vi "Thermal_Camera_Calibration.vi"() -> (2 "State out":string="Data: Load Thermal Calibration")   [LabVIEW 2020]
uses:
  DataCluster_TCAL.ctl
  <vilib>/vision/Image Controls.llb/IMAQ Image.ctl
  DataCluster.ctl
  <vilib>/userdefined/High Color/IMAQdx.ctl
  <vilib>/Utility/xml.llb/Write to XML File(string).vi
panel:
  out "Pict Ring":i32(ring)
  in  "Done":bool
  out "Step":string="Step: 4\n\nCalculate temperature!"
  in  "Fixpoint Radius":i32=20 min=3 max=20
  in  "Cluster":T1 {"PCR Size" items=["384 (24x16)", "96 (12x8)"]; "Points"."Top Left"."Y" format="%.2f"; "Points"."Top Left"."X" format="%.2f"; "Points"."Top Right"."Y" format="%.2f"; "Points"."Top Right"."X" format="%.2f"; "Points"."Bottom Left"."Y" format="%.2f"; "Points"."Bottom Left"."X" format="%.2f"; "Points"."Bottom Right"."Y" format="%.2f"; "Points"."Bottom Right"."X" format="%.2f"; "Points"."Fixpoint"."Y" format="%.2f"; "Points"."Fixpoint"."X" format="%.2f"}
  in  "Display Mapping":u32(ring)=10 items=["Default"=10, "Most Significant Bits"=11, "Full Dynamic"=12, "Downshift"=13, "Given Range"=14, "90% Dynamic"=15, "Given Percent Range"=16]
  in  "Image":u32(slide) scale=0.0..242.0
  in  "Help":bool
  out "Tutorial":string="Step: 4\n\nCalculate temperature!"
  in  "Show All Points":bool
  in  "Well Radius":u32=50 min=1 max=100
  in  "PCR Size":u16(ring) items=["384 (24x16)", "96 (12x8)"]
  out "Points":T3[](array[typedef])=[{"X"=103.0, "Y"=94.0}, {"X"=158.04349, "Y"=93.521736}, {"X"=213.08696, "Y"=93.04348}, {"X"=268.13043, "Y"=92.565216}, {"X"=323.17392, "Y"=92.08696}, {"X"=378.2174, "Y"=91.608696}, {"X"=433.26086, "Y"=91.13043}, {"X"=488.30435, "Y"=90.652176}, {"X"=543.34784, "Y"=90.17391}, {"X"=598.39136, "Y"=89.69565}, {"X"=653.4348, "Y"=89.21739}, {"X"=708.4783, "Y"=88.73913}, {"X"=763.5217, "Y"=88.26087}, {"X"=818.56525, "Y"=87.78261}, {"X"=873.6087, "Y"=87.30435}, {"X"=928.6522, "Y"=86.82609}, {"X"=983.6957, "Y"=86.347824}, {"X"=1038.7391, "Y"=85.86957}, {"X"=1093.7827, "Y"=85.391304}, {"X"=1148.8262, "Y"=84.91304}, {"X"=1203.8696, "Y"=84.434784}, {"X"=1258.9131, "Y"=83.95652}, {"X"=1313.9565, "Y"=83.478264}, {"X"=1369.0, "Y"=83.0}, {"X"=103.46667, "Y"=149.06667}, {"X"=158.51015, "Y"=148.58841}, {"X"=213.55362, "Y"=148.11014}, {"X"=268.5971, "Y"=147.63188}, {"X"=323.6406, "Y"=147.15363}, {"X"=378.68408, "Y"=146.67535}, {"X"=433.72754, "Y"=146.1971}, {"X"=488.77103, "Y"=145.71884}, {"X"=543.8145, "Y"=145.24057}, {"X"=598.858, "Y"=144.76231}, {"X"=653.9015, "Y"=144.28406}, {"X"=708.94495, "Y"=143.8058}, {"X"=763.9884, "Y"=143.32753}, {"X"=819.0319, "Y"=142.84927}, {"X"=874.0754, "Y"=142.37102}, {"X"=929.1189, "Y"=141.89276}, {"X"=984.16235, "Y"=141.41449}, {"X"=1039.2058, "Y"=140.93623}, {"X"=1094.2493, "Y"=140.45798}, {"X"=1149.2928, "Y"=139.9797}, {"X"=1204.3363, "Y"=139.50145}, {"X"=1259.3798, "Y"=139.0232}, {"X"=1314.4232, "Y"=138.54492}, {"X"=1369.4667, "Y"=138.06667}, {"X"=103.933334, "Y"=204.13333}, {"X"=158.9768, "Y"=203.65506}, {"X"=214.0203, "Y"=203.17682}, {"X"=269.06375, "Y"=202.69855}, {"X"=324.10724, "Y"=202.22029}, {"X"=379.15073, "Y"=201.74203}, {"X"=434.19418, "Y"=201.26376}, {"X"=489.23767, "Y"=200.7855}, {"X"=544.2812, "Y"=200.30725}, {"X"=599.32465, "Y"=199.82898}, {"X"=654.36816, "Y"=199.35072}, {"X"=709.4116, "Y"=198.87247}, {"X"=764.4551, "Y"=198.3942}, {"X"=819.4986, "Y"=197.91594}, {"X"=874.54205, "Y"=197.43768}, {"X"=929.5856, "Y"=196.95941}, {"X"=984.629, "Y"=196.48116}, {"X"=1039.6725, "Y"=196.0029}, {"X"=1094.716, "Y"=195.52463}, {"X"=1149.7595, "Y"=195.04637}, {"X"=1204.803, "Y"=194.56812}, {"X"=1259.8464, "Y"=194.08984}, {"X"=1314.8899, "Y"=193.6116}, {"X"=1369.9333, "Y"=193.13333}, {"X"=104.4, "Y"=259.2}, {"X"=159.44348, "Y"=258.72174}, {"X"=214.48695, "Y"=258.24347}, {"X"=269.53043, "Y"=257.7652}, {"X"=324.5739, "Y"=257.28696}, {"X"=379.6174, "Y"=256.8087}, {"X"=434.66086, "Y"=256.33044}, {"X"=489.70435, "Y"=255.85217}, {"X"=544.74786, "Y"=255.37392}, {"X"=599.7913, "Y"=254.89565}, {"X"=654.83484, "Y"=254.41739}, {"X"=709.8783, "Y"=253.93913}, {"X"=764.92175, "Y"=253.46086}, {"X"=819.9653, "Y"=252.9826}, {"X"=875.0087, "Y"=252.50435}, {"X"=930.05225, "Y"=252.02608}, {"X"=985.0957, "Y"=251.54782}, {"X"=1040.1392, "Y"=251.06956}, {"X"=1095.1826, "Y"=250.59131}, {"X"=1150.2262, "Y"=250.11304}, {"X"=1205.2697, "Y"=249.63478}, {"X"=1260.3131, "Y"=249.15652}, {"X"=1315.3566, "Y"=248.67825}, {"X"=1370.4, "Y"=248.2}, {"X"=104.86667, "Y"=314.26666}, {"X"=159.91014, "Y"=313.7884}, {"X"=214.95363, "Y"=313.31012}, {"X"=269.9971, "Y"=312.83188}, {"X"=325.0406, "Y"=312.35364}, {"X"=380.08408, "Y"=311.87537}, {"X"=435.12753, "Y"=311.3971}, {"X"=490.17102, "Y"=310.91882}, {"X"=545.2145, "Y"=310.44058}, {"X"=600.258, "Y"=309.9623}, {"X"=655.30145, "Y"=309.48407}, {"X"=710.3449, "Y"=309.0058}, {"X"=765.38837, "Y"=308.52753}, {"X"=820.4319, "Y"=308.04926}, {"X"=875.47534, "Y"=307.571}, {"X"=930.51886, "Y"=307.09274}, {"X"=985.5623, "Y"=306.6145}, {"X"=1040.6058, "Y"=306.13623}, {"X"=1095.6493, "Y"=305.65796}, {"X"=1150.6929, "Y"=305.1797}, {"X"=1205.7363, "Y"=304.70145}, {"X"=1260.7798, "Y"=304.2232}, {"X"=1315.8232, "Y"=303.74493}, {"X"=1370.8667, "Y"=303.26666}, {"X"=105.333336, "Y"=369.3333}, {"X"=160.37682, "Y"=368.85504}, {"X"=215.42029, "Y"=368.3768}, {"X"=270.46378, "Y"=367.89853}, {"X"=325.50726, "Y"=367.42026}, {"X"=380.55075, "Y"=366.94202}, {"X"=435.5942, "Y"=366.46375}, {"X"=490.6377, "Y"=365.98547}, {"X"=545.68115, "Y"=365.50723}, {"X"=600.7247, "Y"=365.02896}, {"X"=655.7681, "Y"=364.5507}, {"X"=710.8116, "Y"=364.07245}, {"X"=765.85504, "Y"=363.59418}, {"X"=820.89856, "Y"=363.11594}, {"X"=875.942, "Y"=362.63766}, {"X"=930.98553, "Y"=362.1594}, {"X"=986.029, "Y"=361.68115}, {"X"=1041.0725, "Y"=361.20288}, {"X"=1096.116, "Y"=360.7246}, {"X"=1151.1595, "Y"=360.24637}, {"X"=1206.203, "Y"=359.7681}, {"X"=1261.2465, "Y"=359.28983}, {"X"=1316.2899, "Y"=358.81158}, {"X"=1371.3334, "Y"=358.3333}, {"X"=105.8, "Y"=424.4}, {"X"=160.84348, "Y"=423.92172}, {"X"=215.88696, "Y"=423.44348}, {"X"=270.93042, "Y"=422.9652}, {"X"=325.9739, "Y"=422.48694}, {"X"=381.0174, "Y"=422.0087}, {"X"=436.06085, "Y"=421.53043}, {"X"=491.10434, "Y"=421.05215}, {"X"=546.1478, "Y"=420.5739}, {"X"=601.19135, "Y"=420.09564}, {"X"=656.2348, "Y"=419.61737}, {"X"=711.27826, "Y"=419.13913}, {"X"=766.3217, "Y"=418.66086}, {"X"=821.36523, "Y"=418.18262}, {"X"=876.4087, "Y"=417.70435}, {"X"=931.4522, "Y"=417.22607}, {"X"=986.49567, "Y"=416.74783}, {"X"=1041.5392, "Y"=416.26956}, {"X"=1096.5826, "Y"=415.7913}, {"X"=1151.6262, "Y"=415.31305}, {"X"=1206.6697, "Y"=414.83478}, {"X"=1261.7131, "Y"=414.3565}, {"X"=1316.7566, "Y"=413.87827}, {"X"=1371.8, "Y"=413.4}, {"X"=106.26667, "Y"=479.46667}, {"X"=161.31015, "Y"=478.9884}, {"X"=216.35362, "Y"=478.51016}, {"X"=271.3971, "Y"=478.0319}, {"X"=326.44058, "Y"=477.55362}, {"X"=381.48407, "Y"=477.07538}, {"X"=436.52753, "Y"=476.5971}, {"X"=491.571, "Y"=476.11884}, {"X"=546.6145, "Y"=475.6406}, {"X"=601.658, "Y"=475.16232}, {"X"=656.7015, "Y"=474.68405}, {"X"=711.74493, "Y"=474.2058}, {"X"=766.7884, "Y"=473.72754}, {"X"=821.8319, "Y"=473.2493}, {"X"=876.87537, "Y"=472.77103}, {"X"=931.9189, "Y"=472.29276}, {"X"=986.96234, "Y"=471.8145}, {"X"=1042.0059, "Y"=471.33624}, {"X"=1097.0493, "Y"=470.85797}, {"X"=1152.0929, "Y"=470.37973}, {"X"=1207.1364, "Y"=469.90146}, {"X"=1262.1798, "Y"=469.4232}, {"X"=1317.2233, "Y"=468.94495}, {"X"=1372.2667, "Y"=468.46667}, {"X"=106.73333, "Y"=534.5333}, {"X"=161.77681, "Y"=534.05505}, {"X"=216.8203, "Y"=533.5768}, {"X"=271.86377, "Y"=533.0985}, {"X"=326.90726, "Y"=532.62024}, {"X"=381.95074, "Y"=532.142}, {"X"=436.9942, "Y"=531.66376}, {"X"=492.0377, "Y"=531.1855}, {"X"=547.0812, "Y"=530.7073}, {"X"=602.12463, "Y"=530.229}, {"X"=657.16815, "Y"=529.75073}, {"X"=712.2116, "Y"=529.27246}, {"X"=767.25507, "Y"=528.7942}, {"X"=822.2986, "Y"=528.3159}, {"X"=877.34204, "Y"=527.83765}, {"X"=932.38556, "Y"=527.3594}, {"X"=987.429, "Y"=526.88116}, {"X"=1042.4724, "Y"=526.4029}, {"X"=1097.516, "Y"=525.9246}, {"X"=1152.5594, "Y"=525.4464}, {"X"=1207.6029, "Y"=524.96814}, {"X"=1262.6464, "Y"=524.48987}, {"X"=1317.6898, "Y"=524.0116}, {"X"=1372.7333, "Y"=523.5333}, {"X"=107.2, "Y"=589.6}, {"X"=162.24348, "Y"=589.1217}, {"X"=217.28696, "Y"=588.64343}, {"X"=272.33044, "Y"=588.16516}, {"X"=327.37393, "Y"=587.6869}, {"X"=382.41742, "Y"=587.2087}, {"X"=437.46088, "Y"=586.7304}, {"X"=492.50436, "Y"=586.25214}, {"X"=547.54785, "Y"=585.7739}, {"X"=602.5913, "Y"=585.29565}, {"X"=657.6348, "Y"=584.8174}, {"X"=712.6783, "Y"=584.3391}, {"X"=767.72174, "Y"=583.86084}, {"X"=822.76526, "Y"=583.38257}, {"X"=877.8087, "Y"=582.9043}, {"X"=932.85223, "Y"=582.426}, {"X"=987.8957, "Y"=581.9478}, {"X"=1042.9391, "Y"=581.46954}, {"X"=1097.9827, "Y"=580.9913}, {"X"=1153.0261, "Y"=580.51306}, {"X"=1208.0696, "Y"=580.0348}, {"X"=1263.113, "Y"=579.5565}, {"X"=1318.1565, "Y"=579.07825}, {"X"=1373.2, "Y"=578.6}, {"X"=107.666664, "Y"=644.6666}, {"X"=162.71014, "Y"=644.18835}, {"X"=217.75363, "Y"=643.7101}, {"X"=272.7971, "Y"=643.2319}, {"X"=327.84058, "Y"=642.7536}, {"X"=382.88406, "Y"=642.2753}, {"X"=437.92752, "Y"=641.79706}, {"X"=492.971, "Y"=641.3188}, {"X"=548.0145, "Y"=640.8405}, {"X"=603.058, "Y"=640.3623}, {"X"=658.1015, "Y"=639.88403}, {"X"=713.14496, "Y"=639.40576}, {"X"=768.1884, "Y"=638.9275}, {"X"=823.23193, "Y"=638.4492}, {"X"=878.2754, "Y"=637.97095}, {"X"=933.3189, "Y"=637.49274}, {"X"=988.36237, "Y"=637.01447}, {"X"=1043.4058, "Y"=636.5362}, {"X"=1098.4493, "Y"=636.0579}, {"X"=1153.4928, "Y"=635.57965}, {"X"=1208.5363, "Y"=635.1014}, {"X"=1263.5797, "Y"=634.62317}, {"X"=1318.6232, "Y"=634.1449}, {"X"=1373.6666, "Y"=633.6666}, {"X"=108.13333, "Y"=699.73334}, {"X"=163.17682, "Y"=699.25507}, {"X"=218.22029, "Y"=698.7768}, {"X"=273.26376, "Y"=698.2986}, {"X"=328.30725, "Y"=697.8203}, {"X"=383.35074, "Y"=697.34204}, {"X"=438.3942, "Y"=696.8638}, {"X"=493.43768, "Y"=696.3855}, {"X"=548.4812, "Y"=695.9072}, {"X"=603.52466, "Y"=695.429}, {"X"=658.5682, "Y"=694.95074}, {"X"=713.61163, "Y"=694.4725}, {"X"=768.6551, "Y"=693.9942}, {"X"=823.6986, "Y"=693.5159}, {"X"=878.74207, "Y"=693.03766}, {"X"=933.7856, "Y"=692.55945}, {"X"=988.82904, "Y"=692.0812}, {"X"=1043.8724, "Y"=691.6029}, {"X"=1098.916, "Y"=691.12463}, {"X"=1153.9595, "Y"=690.64636}, {"X"=1209.0029, "Y"=690.1681}, {"X"=1264.0464, "Y"=689.6899}, {"X"=1319.0898, "Y"=689.2116}, {"X"=1374.1333, "Y"=688.73334}, {"X"=108.6, "Y"=754.8}, {"X"=163.64348, "Y"=754.3217}, {"X"=218.68697, "Y"=753.84344}, {"X"=273.73044, "Y"=753.36523}, {"X"=328.77393, "Y"=752.88696}, {"X"=383.8174, "Y"=752.4087}, {"X"=438.86087, "Y"=751.9304}, {"X"=493.90436, "Y"=751.45215}, {"X"=548.9478, "Y"=750.9739}, {"X"=603.99133, "Y"=750.49567}, {"X"=659.0348, "Y"=750.0174}, {"X"=714.07825, "Y"=749.5391}, {"X"=769.1217, "Y"=749.06085}, {"X"=824.1652, "Y"=748.5826}, {"X"=879.2087, "Y"=748.1043}, {"X"=934.2522, "Y"=747.6261}, {"X"=989.29565, "Y"=747.1478}, {"X"=1044.3391, "Y"=746.66956}, {"X"=1099.3827, "Y"=746.1913}, {"X"=1154.4261, "Y"=745.713}, {"X"=1209.4696, "Y"=745.23474}, {"X"=1264.5131, "Y"=744.75653}, {"X"=1319.5565, "Y"=744.27826}, {"X"=1374.6, "Y"=743.8}, {"X"=109.066666, "Y"=809.86664}, {"X"=164.11015, "Y"=809.38837}, {"X"=219.15363, "Y"=808.9101}, {"X"=274.1971, "Y"=808.4319}, {"X"=329.2406, "Y"=807.9536}, {"X"=384.2841, "Y"=807.47534}, {"X"=439.32755, "Y"=806.9971}, {"X"=494.37103, "Y"=806.5188}, {"X"=549.4145, "Y"=806.0405}, {"X"=604.458, "Y"=805.5623}, {"X"=659.50146, "Y"=805.08405}, {"X"=714.5449, "Y"=804.6058}, {"X"=769.5884, "Y"=804.1275}, {"X"=824.6319, "Y"=803.64923}, {"X"=879.67535, "Y"=803.17096}, {"X"=934.7189, "Y"=802.69275}, {"X"=989.7623, "Y"=802.2145}, {"X"=1044.8058, "Y"=801.7362}, {"X"=1099.8494, "Y"=801.25793}, {"X"=1154.8928, "Y"=800.77966}, {"X"=1209.9363, "Y"=800.3014}, {"X"=1264.9797, "Y"=799.8232}, {"X"=1320.0232, "Y"=799.3449}, {"X"=1375.0667, "Y"=798.86664}, {"X"=109.53333, "Y"=864.93335}, {"X"=164.57681, "Y"=864.4551}, {"X"=219.6203, "Y"=863.9768}, {"X"=274.66376, "Y"=863.4986}, {"X"=329.70724, "Y"=863.0203}, {"X"=384.75073, "Y"=862.54205}, {"X"=439.7942, "Y"=862.0638}, {"X"=494.83768, "Y"=861.5855}, {"X"=549.88116, "Y"=861.10724}, {"X"=604.9247, "Y"=860.629}, {"X"=659.96814, "Y"=860.15076}, {"X"=715.0116, "Y"=859.6725}, {"X"=770.05505, "Y"=859.1942}, {"X"=825.0986, "Y"=858.71594}, {"X"=880.142, "Y"=858.2377}, {"X"=935.18555, "Y"=857.75946}, {"X"=990.229, "Y"=857.2812}, {"X"=1045.2725, "Y"=856.8029}, {"X"=1100.316, "Y"=856.32465}, {"X"=1155.3595, "Y"=855.8464}, {"X"=1210.403, "Y"=855.3681}, {"X"=1265.4464, "Y"=854.8899}, {"X"=1320.4899, "Y"=854.4116}, {"X"=1375.5333, "Y"=853.93335}, {"X"=110.0, "Y"=920.0}, {"X"=165.04349, "Y"=919.5217}, {"X"=220.08696, "Y"=919.04346}, {"X"=275.13043, "Y"=918.56525}, {"X"=330.17392, "Y"=918.087}, {"X"=385.2174, "Y"=917.6087}, {"X"=440.26086, "Y"=917.13043}, {"X"=495.30435, "Y"=916.65216}, {"X"=550.34784, "Y"=916.1739}, {"X"=605.39136, "Y"=915.6957}, {"X"=660.4348, "Y"=915.2174}, {"X"=715.4783, "Y"=914.73914}, {"X"=770.5217, "Y"=914.26086}, {"X"=825.56525, "Y"=913.7826}, {"X"=880.6087, "Y"=913.3043}, {"X"=935.6522, "Y"=912.8261}, {"X"=990.6957, "Y"=912.34784}, {"X"=1045.7391, "Y"=911.86957}, {"X"=1100.7827, "Y"=911.3913}, {"X"=1155.8262, "Y"=910.913}, {"X"=1210.8696, "Y"=910.43475}, {"X"=1265.9131, "Y"=909.95654}, {"X"=1320.9565, "Y"=909.4783}, {"X"=1376.0, "Y"=909.0}] {"Y" format="%.2f"; "X" format="%.2f"}
  out "State":i32=3
  in  "Previous":bool
  in  "Next":bool
  in  "Path":path caption="Image Path"
  out "Image":T2(plugin-control)
  # "hints \nPress F1 or F2 to cycle through the steps\nUse the Mouse Wheel to zoom in and out"
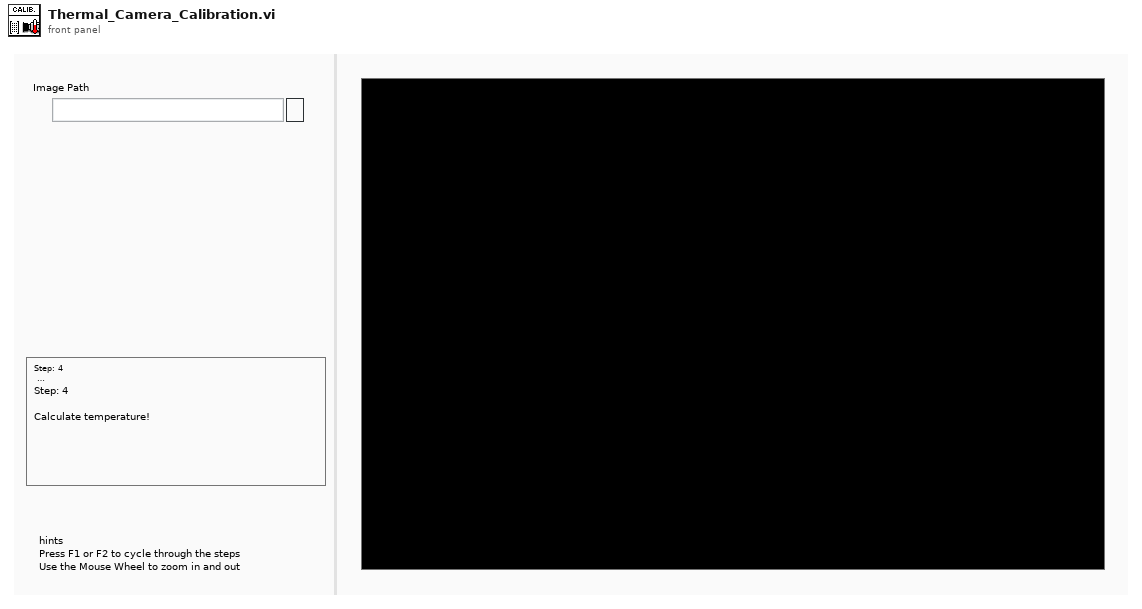
[diagram p1: front panel]
types:
  T1 = typedef "DataCluster_TCAL.ctl" = cluster{"Core":cluster{"Current VI Reference":refnum<vi>, "Close Panel on Exit?":bool}, "Image Out":T2, "State":i32, "Points":cluster{"Top Left":T3, "Top Right":T3, "Bottom Left":T3, "Bottom Right":T3, "x space 2":dbl, "y space 2":sgl, "x_space":sgl, "y_space":sgl, "Pixels":cluster{"X":i32, "Y":i32}[][], "Fixpoint":T3}, "img_array":T2[], "Temps":dbl[], "Temps_Array":dbl[][], "Scan Area":dbl, "Fixpoint Area":dbl, "PCR Size":u16}
  T2 = typedef "IMAQ Image.ctl" = refnum<image>
  T3 = typedef "IMAQ Point" = cluster{"X":sgl, "Y":sgl}
  T4 = enum32{"Invalid", "Standard", "Closed", "Hidden", "Minimized", "Maximized"}
  T5 = enum32{"invalid app kind", "Development System", "Run Time System", "Student Edition", "Embedded LabVIEW", "Evaluation", "Custom"}
  T6 = cluster{"Global Rectangle":i32[], "Contours":cluster{"Contour Type":u32, "ROI Type":u32, "Points":i32[]}[]}
  T7 = typedef "DataCluster.ctl" = cluster{"Core":cluster{"Current VI Reference":refnum<vi>, "Close Panel on Exit?":bool, "Exit":bool, "Initialized?":bool}, "Connections":cluster{"cDAQ Therm":cluster{"Task":refnum<k21>, "Connected":bool, "Active":bool}, "cDAQ Voltage":cluster{"Task":refnum<k21>, "Connected":bool, "Active":bool}, "cDAQ ID":string, "Camera":cluster{"Session":T8, "Connected":bool, "Active":bool, "Placeholder":T2}, "PSU":cluster{"Port":refnum<visa-resource-name>, "Connected":bool, "Active":bool}}, "Data Acquisition":cluster{"Setup":cluster{"Label":string, "Operator":string, "Notes":string, "TempGrad":dbl, "TargetTemp":dbl, "Sample Volume":dbl}, "Camera":cluster{"Image":T2, "Save Image":T2, "Image Frequency":i32, "Rectangle":T9, "Calibration":cluster{"Top Left":T3, "Top Right":T3, "Bottom Left":T3, "Bottom Right":T3, "Fixpoint":T3, "Scan Area":dbl, "Fixpoint Area":dbl, "Well Pixels":cluster{"X":i32, "Y":i32}[][], "Valid":bool}, "FocusPos":u32, "Display Mapping":u32}, "Thermistor":cluster{"Sample Size":i32, "Calibration":cluster{"B0.100":dbl[], "R25":dbl[], "c":dbl[][], "State":bool[], "V_S":dbl, "R_S":dbl}, "Timing Mode":i32}, "Partition":cluster{"Data":string[][], "Cell Label":string, "Cell Color":u32, "Height":i32, "Width":i32, "Grid":string[][]}, "Queue":cluster{"Size":i32, "Queue":refnum<queue>}, "Sample Rate":i32, "Active":bool, "Ready":bool, "Graph Mode":u16}, "Control":cluster{"Sample Rate":i32, "PID gains":cluster{"proportional gain (Kc)":dbl, "integral time (Ti, min)":dbl, "derivative time (Td, min)":dbl}}}
  T8 = typedef "IMAQdx.ctl" = refnum<k21>
  T9 = typedef "IMAQ Rectangle" = cluster{"Left":i32, "Top":i32, "Right":i32, "Bottom":i32, "Rotation":dbl}
  T10 = enum16{"open", "replace", "create", "open or create", "replace or create", "replace or create with confirmation"}
  T11 = typedef "ROI Descriptor" = cluster{"Global Rectangle":i32[], "Contours":cluster{"ID":enum32{"External", "Internal"}, "Type":u32, "Coordinates":i32[]}[]}
  T12 = typedef "Image Type" = u32
  T13 = cluster{"Current VI Reference":refnum<vi>, "Close Panel on Exit?":bool}
  T14 = cluster{"Top Left":T3, "Top Right":T3, "Bottom Left":T3, "Bottom Right":T3, "x space 2":dbl, "y space 2":sgl, "x_space":sgl, "y_space":sgl, "Pixels":cluster{"X":i32, "Y":i32}[][], "Fixpoint":T3}
  T15 = cluster{"Top Left":T3, "Top Right":T3, "Bottom Left":T3, "Bottom Right":T3, "Fixpoint":T3, "Scan Area":dbl, "Fixpoint Area":dbl, "Well Pixels":cluster{"X":i32, "Y":i32}[][], "Valid":bool}
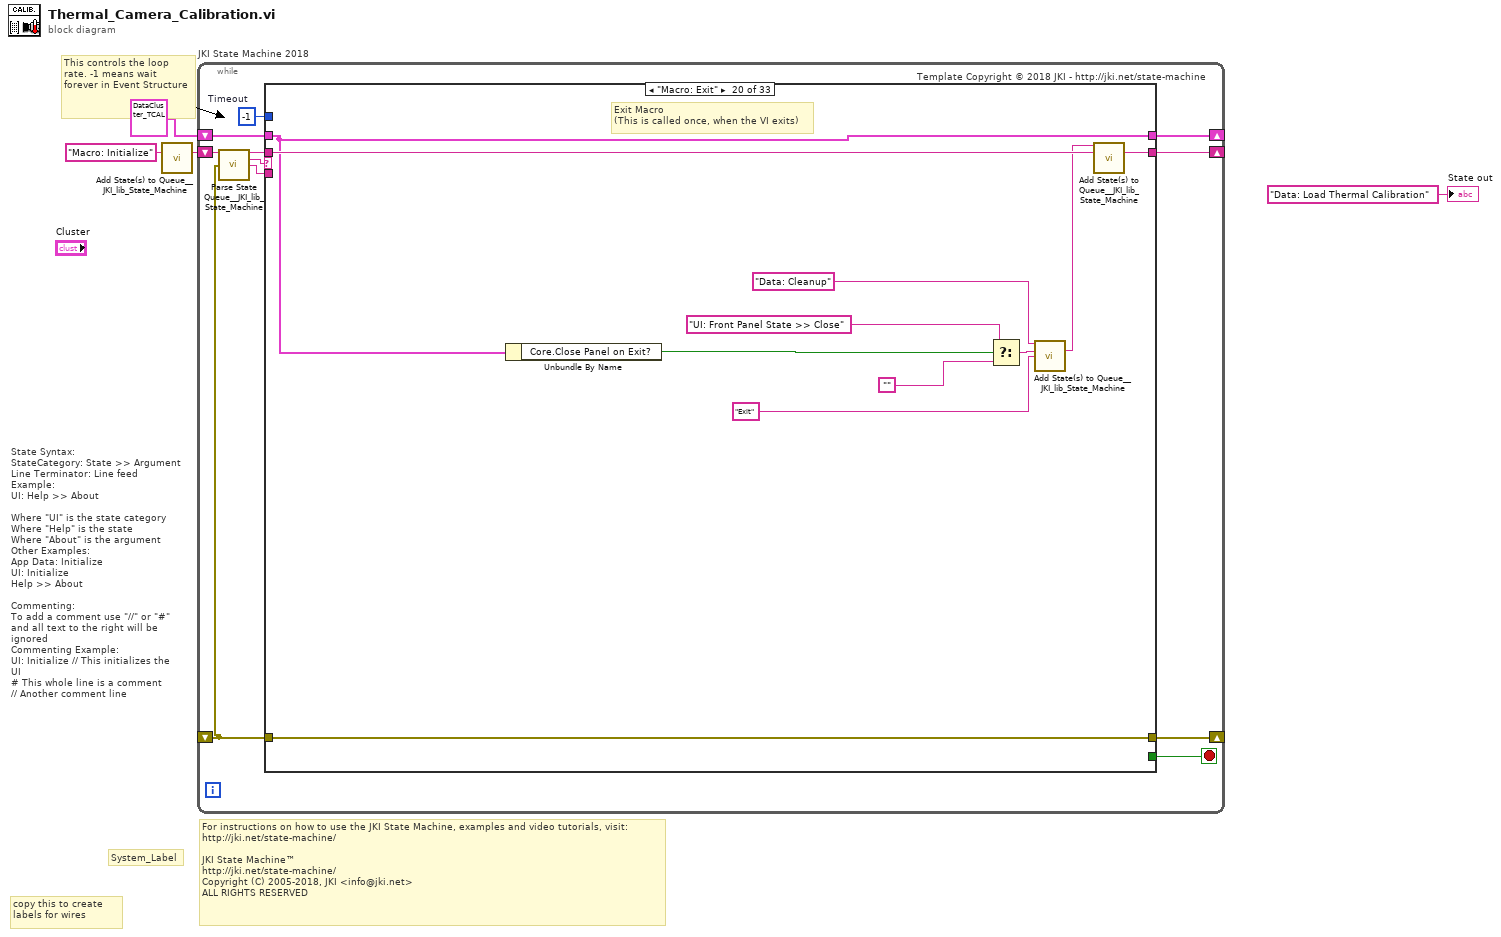
[diagram p0: block diagram]
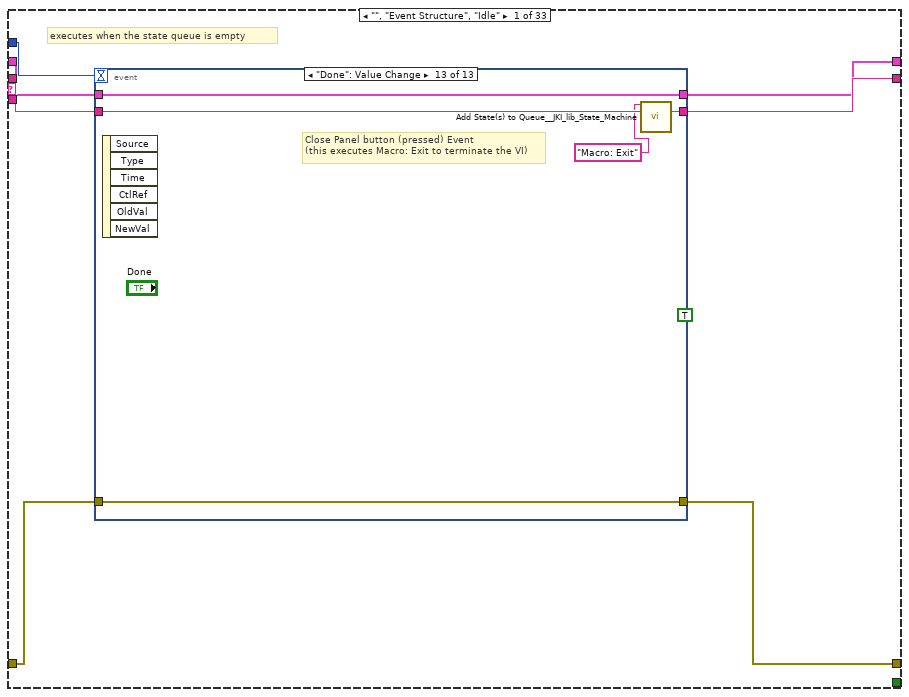
[diagram p2: hidden frame]
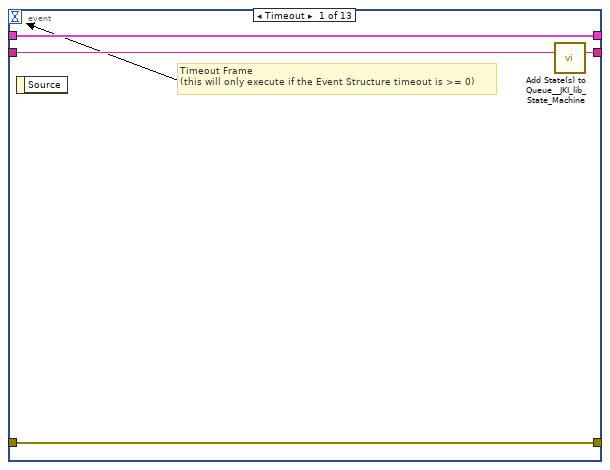
[diagram p3: hidden frame]
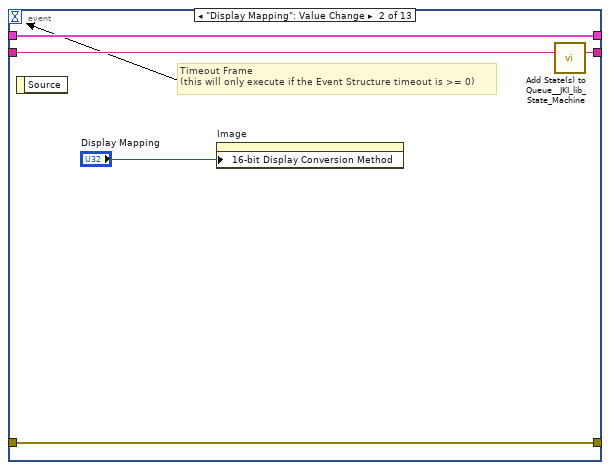
[diagram p4: hidden frame]
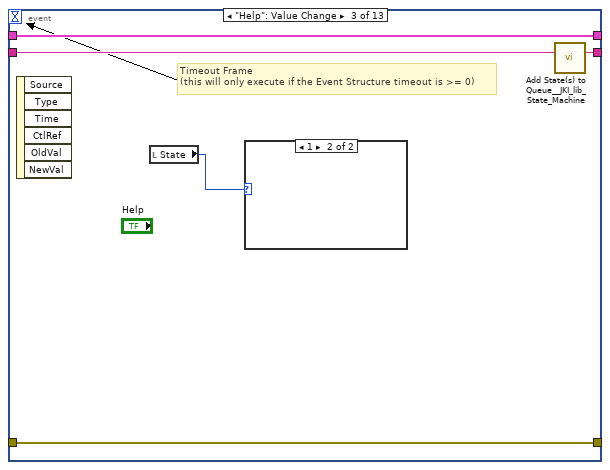
[diagram p5: hidden frame]
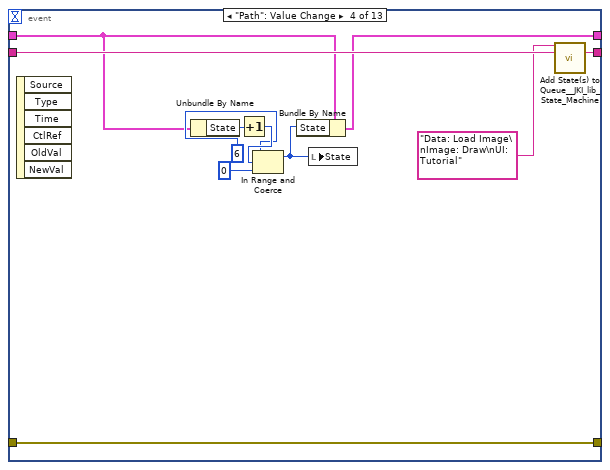
[diagram p7: hidden frame]
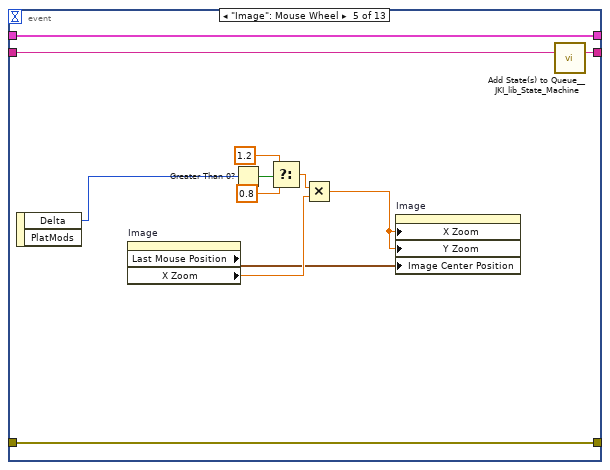
[diagram p8: hidden frame]
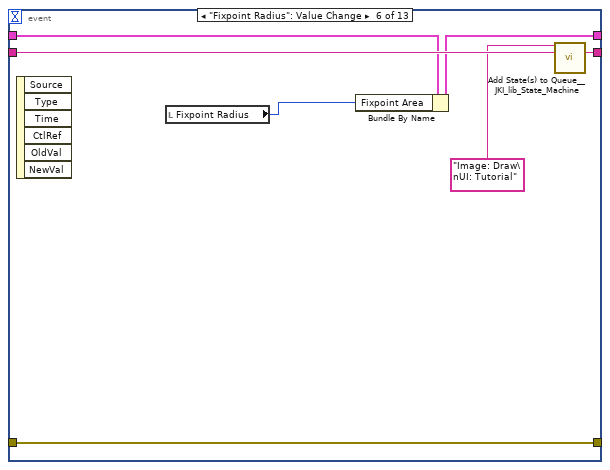
[diagram p9: hidden frame]
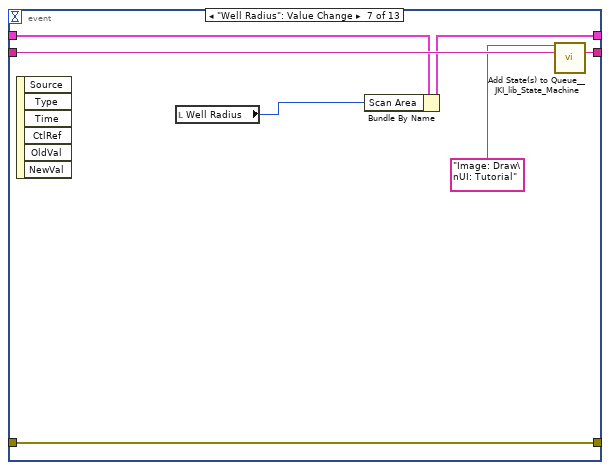
[diagram p10: hidden frame]
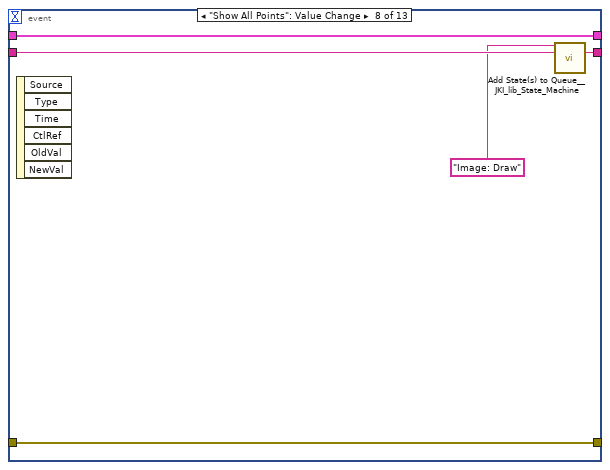
[diagram p11: hidden frame]
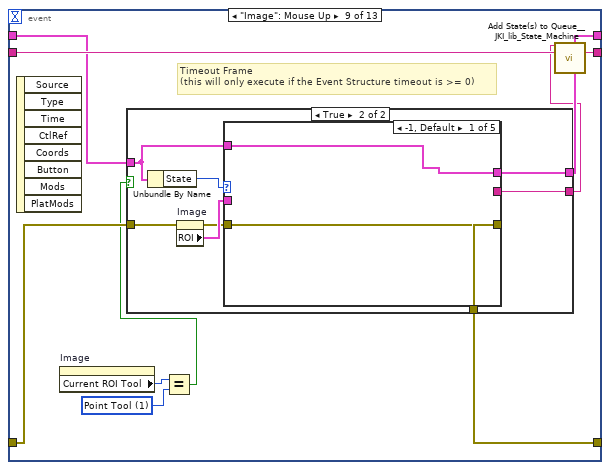
[diagram p12: hidden frame]
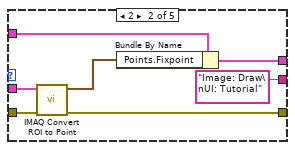
[diagram p14: hidden frame]
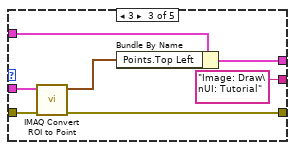
[diagram p15: hidden frame]
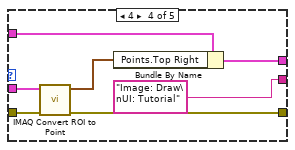
[diagram p16: hidden frame]
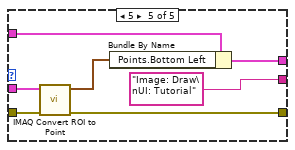
[diagram p17: hidden frame]
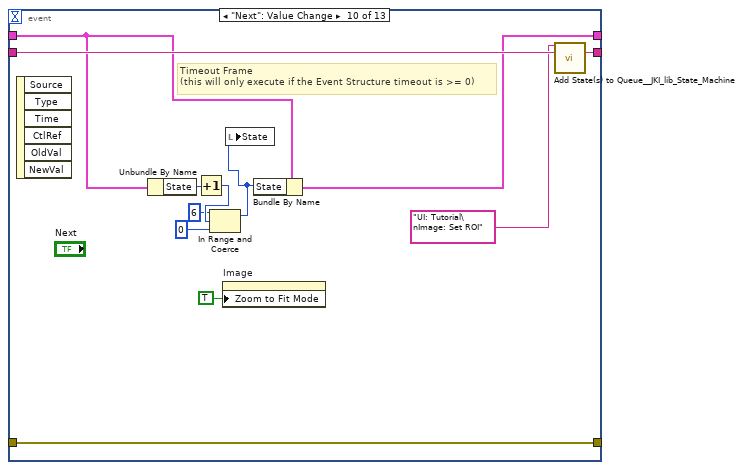
[diagram p18: hidden frame]
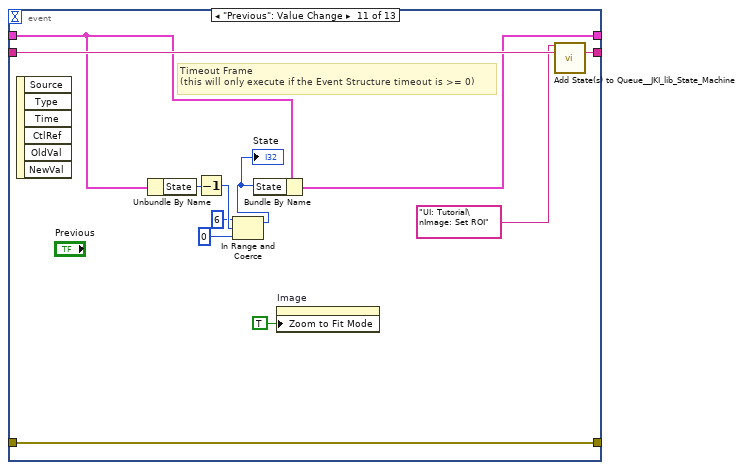
[diagram p19: hidden frame]
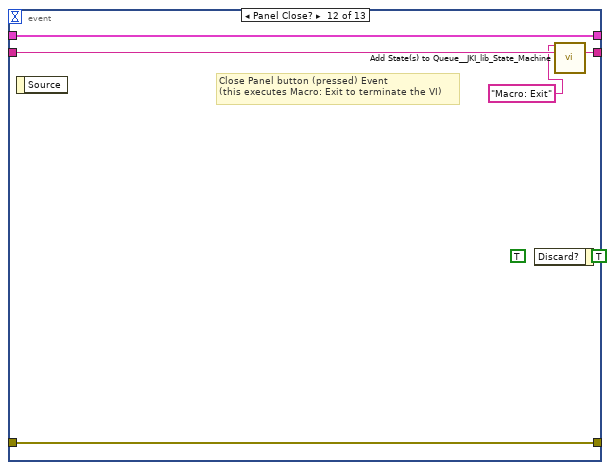
[diagram p20: hidden frame]
diagram:
  # "For instructions on how to use the JKI State Machine, examples and video tutorials, visit:\nhttp://jki.net/state-machine/\n\nJKI State Machine™\nhttp://jki.net/state-machine/\nCopyright (C) 2005-2018, JKI <info@jki.net>\nALL RIGHTS RESERVED"
  # "State Syntax:\nStateCategory: State >> Argument\nLine Terminator: Line feed\nExample:\nUI: Help >> About\n\nWhere \"UI\" is the state category\nWhere \"Help\" is the state\nWhere \"About\" is the argument\nOther Examples:\nApp Data: Initialize\nUI: Initialize\nHelp >> About\n\nCommenting:\nTo add a comment use \"//\" or \"#\" and all text to the right will be ignored\nCommenting Example:\nUI: Initialize // This initializes the UI\n# This whole line is a comment\n// Another comment line"
  # "copy this to create labels for wires"
  # "This controls the loop rate. -1 means wait forever in Event Structure"
  # "System_Label"
  n1 = call <vilib>:"Add State(s) to Queue__JKI_lib_State_Machine.vi"("State(s) in (\"\")"="Macro: Initialize") -> ("States Out"=w4:string)  [unwired: 14 in]
  n2 = while "JKI State Machine 2018" {
    shift-right: [w8] -> _
    shift-left: T1 {"Core"={"Current VI Reference"=refnum, "Close Panel on Exit?"=FALSE}, "Image Out"=refnum, "State"=0, "Points"={"Top Left"={"X"=0.0, "Y"=0.0}, "Top Right"={"X"=0.0, "Y"=0.0}, "Bottom Left"={"X"=0.0, "Y"=0.0}, "Bottom Right"={"X"=0.0, "Y"=0.0}, "x space 2"=0.0, "y space 2"=0.0, "x_space"=0.0, "y_space"=0.0, "Pixels"=[], "Fixpoint"={"X"=0.0, "Y"=0.0}}, "img_array"=[], "Temps"=[], "Temps_Array"=[], "Scan Area"=0.0, "Fixpoint Area"=0.0, "PCR Size"=0} ("output cluster") -> [w7]
    shift-right: [w11] -> _
    shift-left: _ -> [w5]
    shift-right: [w10] -> _
    shift-left: w4 -> [w12]
    stop <- w9 stop-if-true
    w6 = -1  # Timeout
    # "Template Copyright © 2018 JKI - http://jki.net/state-machine"
    n3 = call <vilib>:"Parse State Queue__JKI_lib_State_Machine.vi"("State Queue"=w12, "Error In (no error)"=w5) -> ("Remaining States"=w14:string, "Current State"=w15:string, "Arguments"=w13:string)  [unwired: 11 in]
    n4 = case shown="\"Macro: Exit\"" w15 {
      selector: w15 -> [_ _ w168 _ _ _ _ _ _ _ _ _ _ _ _ _ _ _ _ _ _ _ _ _ _ _ _ _ _ _ _ _ _]
      tunnel: w14 -> [w22 w167 w172 w191 w197 w202 w206 w215 w236 w241 w256 w289 w299 w319 w337 w398 w409 w478 w483 w494 w498 w503 w508 w528 w545 w551 w569 w589 w607 w618 w646 w711 w733]
      tunnel: w13 -> [_ _ _ _ _ _ _ _ _ _ _ _ _ _ _ w393 w403 _ _ _ _ _ _ _ _ _ _ _ _ _ w644 _ _]
      tunnel: w7 -> [w20 w164 w170 w184 w194 w200 w203 w213 w233 w237 _ w286 w296 w317 w324 w396 w405 w475 w480 w491 w495 w500 w505 w509 w543 w549 w560 w580 w598 w616 w642 w698 w722]
      tunnel: [w19 w165 w174 w188 errorcluster {"status"=FALSE, "code"=0, "source"=""} ("error out") w199 w204 w207 w230 w239 w247 w283 w297 w316 w335 w394 w406 w476 w481 w492 w496 w501 w506 w526 w538 w546 w567 w587 w605 w611 w639 w708 w731] -> w11
      tunnel: w5 -> [w18 w165 w173 w188 w193 w199 w204 w211 w230 w239 w248 w271 w297 w316 w335 w395 w407 w476 w481 w492 w496 w501 w506 w526 w538 w547 w567 w587 w605 w615 w640 w708 w731]
      tunnel: [w21 w166 w171 w190 w196 w201 w205 w214 w235 w240 w255 w288 w298 w318 w336 w397 w408 w477 w482 w493 w497 w502 w507 w527 w544 w550 w568 w588 w606 w617 w645 w710 w732] -> w10
      tunnel: [_ _ _ _ _ TRUE _ _ _ _ _ _ _ _ _ _ _ _ _ _ _ _ _ _ _ _ _ _ _ _ _ _ _] -> w9
      tunnel: [w17 w164 w170 w189 w194 w200 w203 w212 w234 w237 w254 w286 w296 w317 w324 w396 w405 w475 w480 w491 w495 w500 w505 w509 w543 w549 w559 w579 w597 w616 w642 w697 w722] -> w8
      tunnel: w6 -> [w16 _ _ _ _ _ _ _ _ _ _ _ _ _ _ _ _ _ _ _ _ _ _ _ _ _ _ _ _ _ _ _ _]
      frame "", "Event Structure", "Idle" {
        # "executes when the state queue is empty"
        n5 = event shown="[12] \"Done\": Value Change" {
          selector: _ -> [_ _ _ _ _ _ _ _ _ _ _ _ _]
          dyn-events: _ -> [_ _ _ _ _ _ _ _ _ _ _ _ _]
          timeout: w16 -> [_ _ _ _ _ _ _ _ _ _ _ _ _]
          tunnel: w22 -> [w26 w31 w36 w47 w59 w66 w73 w78 w88 w140 w152 w158 w163]
          tunnel: [w25 w30 w35 w46 w58 w65 w72 w77 w87 w139 w151 w157 w162] -> w21
          tunnel: w20 -> [w23 w28 w33 w38 w56 w63 w70 w75 w85 w138 w150 w155 w160]
          tunnel: [w24 w29 w34 w45 w57 w64 w71 w76 w83 w135 w147 w156 w161] -> w19
          tunnel: w18 -> [w24 w29 w34 w45 w57 w64 w71 w76 w86 w135 w147 w156 w161]
          tunnel: [w23 w28 w33 w39 w56 w61 w68 w75 w84 w136 w148 w155 w160] -> w17
          event Timeout {
            # "Timeout Frame\n(this will only execute if the Event Structure timeout is >= 0)"
            n6 = event-data() -> ()  [unwired: 1 in, 1 out]
            n7 = call <vilib>:"Add State(s) to Queue__JKI_lib_State_Machine.vi"("State(s) in (\"\")"=w26) -> ("States Out"=w25:string)  [unwired: 14 in]
          }
          event "Display Mapping": Value Change {
            # "Timeout Frame\n(this will only execute if the Event Structure timeout is >= 0)"
            n8 = event-data() -> ()  [unwired: 1 in, 1 out]
            n9 = property on="Image" class="ImageControl"("16-bit Display Conversion Method"="Display Mapping") -> ()  [unwired: 2 in, 2 out]
            n10 = call <vilib>:"Add State(s) to Queue__JKI_lib_State_Machine.vi"("State(s) in (\"\")"=w31) -> ("States Out"=w30:string)  [unwired: 14 in]
          }
          event "Help": Value Change {
            # "Timeout Frame\n(this will only execute if the Event Structure timeout is >= 0)"
            n11 = event-data() -> ()  [unwired: 1 in, 6 out]
            n12 = local read "State"() -> (w32:i32)
            n13 = case shown="1" w32 {
              frame 0, Default {
              }
              frame 1 {
              }
            }
            n14 = call <vilib>:"Add State(s) to Queue__JKI_lib_State_Machine.vi"("State(s) in (\"\")"=w36) -> ("States Out"=w35:string)  [unwired: 14 in]
          }
          event "Path": Value Change {
            n15 = event-data() -> ()  [unwired: 1 in, 6 out]
            n16 = Unbundle By Name(w38) -> ("State"=w43:i32)
            n17 = Increment(x=w43) -> (x+1=w42:i32)
            n18 = In Range and Coerce(upper limit=6, x=w42, lower limit=0) -> (coerced(x)=w37:i32)  [unwired: 1 out]
            n19 = Bundle By Name(cluster=w38, "State"=w37) -> (w39:T1)
            n20 = local write "State"(w37) -> ()
            n21 = call <vilib>:"Add State(s) to Queue__JKI_lib_State_Machine.vi"("State(s) in Front (\"\")"="Data: Load Image\nImage: Draw\nUI: Tutorial" ("State(s) in Front (\"\")"), "State(s) in (\"\")"=w47) -> ("States Out"=w46:string)  [unwired: 13 in]
          }
          event "Image": Mouse Wheel {
            n22 = event-data() -> ("Delta"=w55:i32)  [unwired: 1 in, 1 out]
            n23 = property on="Image" class="ImageControl"() -> ("Last Mouse Position"=w49:cluster{"X":i32, "Y":i32}, "X Zoom"=w50:sgl)  [unwired: 2 in, 2 out]
            n24 = Greater Than 0?(x=w55) -> (x > 0?=w54:bool)
            n25 = Select(t=1.2, s=w54, f=0.8) -> (s? t:f=w51:dbl)
            n26 = Multiply(x=w51, y=w50) -> (x*y=w48:dbl)
            n27 = property on="Image" class="ImageControl"("X Zoom"=w48, "Y Zoom"=w48, "Image Center Position"=w49) -> ()  [unwired: 2 in, 2 out]
            n28 = call <vilib>:"Add State(s) to Queue__JKI_lib_State_Machine.vi"("State(s) in (\"\")"=w59) -> ("States Out"=w58:string)  [unwired: 14 in]
          }
          event "Fixpoint Radius": Value Change {
            n29 = event-data() -> ()  [unwired: 1 in, 6 out]
            n30 = local read "Fixpoint Radius"() -> (w60:i32)
            n31 = Bundle By Name(cluster=w63, "Fixpoint Area"=w60) -> (w61:T1)
            n32 = call <vilib>:"Add State(s) to Queue__JKI_lib_State_Machine.vi"("State(s) in Front (\"\")"="Image: Draw\nUI: Tutorial" ("State(s) in Front (\"\")"), "State(s) in (\"\")"=w66) -> ("States Out"=w65:string)  [unwired: 13 in]
          }
          event "Well Radius": Value Change {
            n33 = event-data() -> ()  [unwired: 1 in, 6 out]
            n34 = local read "Well Radius"() -> (w67:u32)
            n35 = Bundle By Name(cluster=w70, "Scan Area"=w67) -> (w68:T1)
            n36 = call <vilib>:"Add State(s) to Queue__JKI_lib_State_Machine.vi"("State(s) in Front (\"\")"="Image: Draw\nUI: Tutorial" ("State(s) in Front (\"\")"), "State(s) in (\"\")"=w73) -> ("States Out"=w72:string)  [unwired: 13 in]
          }
          event "Show All Points": Value Change {
            n37 = event-data() -> ()  [unwired: 1 in, 6 out]
            n38 = call <vilib>:"Add State(s) to Queue__JKI_lib_State_Machine.vi"("State(s) in Front (\"\")"="Image: Draw" ("State(s) in Front (\"\")"), "State(s) in (\"\")"=w78) -> ("States Out"=w77:string)  [unwired: 13 in]
          }
          event "Image": Mouse Up {
            w81 = u32 1 items=["Zoom Tool"=8, "Selection Tool"=0, "Pan Tool"=9, "Point Tool"=1, "Line Tool"=2, "Rectangle Tool"=3, "Rotated Rectangle Tool"=12, "Polyline Tool"=10, "Polygon Tool"=5, "Freehand Tool"=11, "Closed Freehand Tool"=6, "Ellipse Tool"=4, "Annulus Tool"=7] ("Current ROI Tool")
            # "Timeout Frame\n(this will only execute if the Event Structure timeout is >= 0)"
            n39 = event-data() -> ()  [unwired: 1 in, 8 out]
            n40 = property on="Image" class="ImageControl"() -> ("Current ROI Tool"=w82:u32)  [unwired: 2 in, 2 out]
            n41 = Equal?(x=w82, y=w81) -> (x = y?=w80:bool)
            n42 = case shown="True" w80 {
              tunnel: w86 -> [w90 w95]
              tunnel: w85 -> [w89 w94]
              tunnel: [w89 w93] -> w84
              tunnel: [w90 w92] -> w83
              tunnel: [_ w91] -> w79
              frame False {
              }
              frame True {
                n43 = Unbundle By Name(w94) -> ("State"=w98:i32)
                n44 = property on="Image" class="ImageControl"(error in=w95) -> (error out=w96:errorcluster, "ROI"=w97:T6)  [unwired: 1 in, 1 out]
                n45 = case shown="-1, Default" w98 {
                  tunnel: w97 -> [_ w106 w113 w121 w128]
                  tunnel: w96 -> [w99 w105 w112 w120 w127]
                  tunnel: w94 -> [w100 w102 w109 w119 w126]
                  tunnel: [w100 w103 w110 w118 w125] -> w93
                  tunnel: [w99 w104 w111 w116 w123] -> w92
                  tunnel: [_ "Image: Draw\nUI: Tutorial" "Image: Draw\nUI: Tutorial" "Image: Draw\nUI: Tutorial" "Image: Draw\nUI: Tutorial"] -> w91
                  frame -1, Default {
                  }
                  frame 2 {
                    n46 = call "IMAQ Convert ROI to Point"("error in (no error)"=w105, "ROI Descriptor"=w106) -> ("error out"=w104:errorcluster, "Point"=w107:T3)  [unwired: 7 in]
                    n47 = Bundle By Name(cluster=w102, "Points.Fixpoint"=w107) -> (w103:T1)
                  }
                  frame 3 {
                    n48 = call "IMAQ Convert ROI to Point"("error in (no error)"=w112, "ROI Descriptor"=w113) -> ("error out"=w111:errorcluster, "Point"=w114:T3)  [unwired: 7 in]
                    n49 = Bundle By Name(cluster=w109, "Points.Top Left"=w114) -> (w110:T1)
                  }
                  frame 4 {
                    n50 = call "IMAQ Convert ROI to Point"("error in (no error)"=w120, "ROI Descriptor"=w121) -> ("error out"=w116:errorcluster, "Point"=w117:T3)  [unwired: 7 in]
                    n51 = Bundle By Name(cluster=w119, "Points.Top Right"=w117) -> (w118:T1)
                  }
                  frame 5 {
                    n52 = call "IMAQ Convert ROI to Point"("error in (no error)"=w127, "ROI Descriptor"=w128) -> ("error out"=w123:errorcluster, "Point"=w124:T3)  [unwired: 7 in]
                    n53 = Bundle By Name(cluster=w126, "Points.Bottom Left"=w124) -> (w125:T1)
                  }
                }
              }
            }
            n54 = call <vilib>:"Add State(s) to Queue__JKI_lib_State_Machine.vi"("State(s) in Front (\"\")"=w79, "State(s) in (\"\")"=w88) -> ("States Out"=w87:string)  [unwired: 13 in]
          }
          event "Next": Value Change {
            # "Timeout Frame\n(this will only execute if the Event Structure timeout is >= 0)"
            n55 = event-data() -> ()  [unwired: 1 in, 6 out]
            n56 = Unbundle By Name(w138) -> ("State"=w137:i32)
            n57 = Increment(x=w137) -> (x+1=w133:i32)
            n58 = In Range and Coerce(upper limit=6, x=w133, lower limit=0) -> (coerced(x)=w130:i32)  [unwired: 1 out]
            n59 = property on="Image" class="ImageControl"("Zoom to Fit Mode"=TRUE) -> ()  [unwired: 2 in, 2 out]
            n60 = local write "State"(w130) -> ()
            n61 = Bundle By Name(cluster=w138, "State"=w130) -> (w136:T1)
            n62 = call <vilib>:"Add State(s) to Queue__JKI_lib_State_Machine.vi"("State(s) in Front (\"\")"="UI: Tutorial\nImage: Set ROI" ("f"), "State(s) in (\"\")"=w140) -> ("States Out"=w139:string)  [unwired: 13 in]
          }
          event "Previous": Value Change {
            # "Timeout Frame\n(this will only execute if the Event Structure timeout is >= 0)"
            n63 = event-data() -> ()  [unwired: 1 in, 6 out]
            n64 = Unbundle By Name(w150) -> ("State"=w149:i32)
            n65 = Decrement(x=w149) -> (x-1=w144:i32)
            n66 = In Range and Coerce(upper limit=6, x=w144, lower limit=0) -> (coerced(x)=w145:i32)  [unwired: 1 out]
            "State" <- w145
            n67 = Bundle By Name(cluster=w150, "State"=w145) -> (w148:T1)
            n68 = property on="Image" class="ImageControl"("Zoom to Fit Mode"=TRUE) -> ()  [unwired: 2 in, 2 out]
            n69 = call <vilib>:"Add State(s) to Queue__JKI_lib_State_Machine.vi"("State(s) in Front (\"\")"="UI: Tutorial\nImage: Set ROI" ("f"), "State(s) in (\"\")"=w152) -> ("States Out"=w151:string)  [unwired: 13 in]
          }
          event Panel Close? {
            (unwired) TRUE ("Discard?")
            # "Close Panel button (pressed) Event\n(this executes Macro: Exit to terminate the VI)"
            n70 = event-data() -> ()  [unwired: 1 in, 1 out]
            n71 = event-data("Discard?"=TRUE) -> ()  [unwired: 1 in, 1 out]
            n72 = call <vilib>:"Add State(s) to Queue__JKI_lib_State_Machine.vi"("State(s) in Front (\"\")"="Macro: Exit", "State(s) in (\"\")"=w158) -> ("States Out"=w157:string)  [unwired: 13 in]
          }
          event "Done": Value Change {
            (unwired) TRUE ("Discard?")
            # "Close Panel button (pressed) Event\n(this executes Macro: Exit to terminate the VI)"
            n73 = event-data() -> ()  [unwired: 1 in, 6 out]
            n74 = call <vilib>:"Add State(s) to Queue__JKI_lib_State_Machine.vi"("State(s) in Front (\"\")"="Macro: Exit", "State(s) in (\"\")"=w163) -> ("States Out"=w162:string)  [unwired: 13 in]
          }
        }
      }
      frame "---------- Core ----------" {
        # "Do not put any code in this frame.\n(it is a separator no-op)"
        n75 = call <vilib>:"Add State(s) to Queue__JKI_lib_State_Machine.vi"("State(s) in (\"\")"=w167) -> ("States Out"=w166:string)  [unwired: 14 in]
      }
      frame Default {
        w177 = 42 items=["No error", "Argument error", "Memory is full", "Out of zone", "End of file", "File already open", "Generic file I/O error", "File not found", "File permission error", "Disk is full", "Duplicate path", "Too many files open", "System feature not enabled", "Resource file not found", "Cannot add resource", "Resource not found", "Image not found", "Image memory error", "Pen does not exist", "Config type invalid", "Config token not found", "Config parse error", "Config memory error", "Bad external code format", "Bad external code offset", "External code not present", "Null window", "Destroy window error", "Null menu", "Print aborted", "Bad print record", "Print driver error", "Windows error during printing", "Memory error during printing", "Print dialog error", "Generic print error", "Invalid device refnum", "Device not found", "Device parameter error", "Device unit error", "Cannot open device", "Device call aborted", "Generic error", "Cancelled by user", "Object ID too low", "Object ID too high", "Object not in heap", "Unknown heap", "Unknown object (invalid DefProc)", "Unknown object (DefProc not in table)", "Message out of range", "Invalid (null) method", "Unknown message", "Manager call not supported", "Bad address", "Network operation in progress", "Network operation timed out", "Connection is busy", "Network attribute not supported", "Network error", "Address in use", "System out of memory", "Connection aborted", "Connection refused", "Not connected", "Already connected", "Connection closed", "Initialization error (interapplication manager)", "Bad occurrence", "Wait on unbound occurrence handler", "Occurrence queue overflow", "Datalog type conflict", "Unused", "Unrecognized type (interapplication manager)", "Memory corrupt", "Failed to make temporary DLL", "Old CIN version", "Drag socket not found", "Failed to load drop-object", "Failed to register OLE object", "Failed to release OLE object", "Format specifier type mismatch", "Unknown format specifier", "Too few format specifiers", "Too many format specifiers", "Scan failed", "Newer CIN version", "Error converting to variant", "Runtime menu error", "Password tampered", "Variant attribute not found", "Incompatible variant data type", "Event data is not available", "Event Store is not present", "Occurrence is not found", "Event Queue is not created", "Event info is not available", "Refnum passed is NULL", "Error retrieving Class GUID", "Error retrieving CoClass GUID", "Error retrieving TypeLib GUID.", "Bad built application magic bytes.", "Specific driver is different from the specific driver associated with the Logical Name.", "There is no session opened to the class driver.", "Max Error", "MAX - Error with config objects", "MAX - Error loading configuration", "MAX - Group not supported"]
        # "Current State"
        # "Do not delete, rename, or modify this frame.\n(this is used to capture unhandled states and typos)"
        # "Handle mistyped state name (developer tool)"
        n76 = Format Into String(format string="Software Exception: Unhandled State \"%s\"." ("message"), error in=w173, w168) -> (resulting string=w176:string, error out=w175:errorcluster)  [unwired: 1 in]
        n77 = call <vilib>:"Error Cluster From Error Code.vi"("show call chain? (False)"=TRUE, "error in (no error)"=w175, "error message (\"\")"=w176, "error code (0)"=w177) -> ("error out"=w174:errorcluster)  [unwired: 5 in]
        n78 = call <vilib>:"Add State(s) to Queue__JKI_lib_State_Machine.vi"("State(s) in (\"\")"=w172) -> ("States Out"=w171:string)  [unwired: 14 in]
      }
      frame "Initialize Core Data" {
        # "Do not delete, rename, or modify this frame.\n(this is used to determine panel behavior on exit)"
        # "originally closed?"
        # "exe?"
        # "If panel starts closed or is an EXE, then close it when we exit"
        n79 = property class="App"() -> ("App.Kind"=w187:T5)  [unwired: 2 in, 2 out]
        n80 = control-ref of="Current VI Reference"() -> (w182:refnum<vi>)
        n81 = property class="VI"() -> ("FP.State"=w181:T4)  [unwired: 2 in, 2 out]
        n82 = Equal?(x=w181, y=T4."Closed" ("Front Panel Window:State")) -> (x = y?=w179:bool)
        n83 = Equal?(x=w187, y=T5."Run Time System" ("Application:Kind")) -> (x = y?=w185:bool)
        n84 = Or(x=w179, y=w185) -> (x .or. y?=w183:bool)
        n85 = Bundle By Name(cluster=w184, "Core.Current VI Reference"=w182, "Core.Close Panel on Exit?"=w183) -> (w189:T1)
        n86 = call <vilib>:"Add State(s) to Queue__JKI_lib_State_Machine.vi"("State(s) in (\"\")"=w191) -> ("States Out"=w190:string)  [unwired: 14 in]
      }
      frame "Error Handler" {
        # "Unhandled Error -- Display it"
        # "Handle any errors here.\nYou can also output any states to clean-up after errors occur"
        # "Clear error"
        n87 = call <vilib>:"General Error Handler.vi"("error in (no error)"=w193) -> ()  [unwired: 10 in, 5 out]
        n88 = call <vilib>:"Add State(s) to Queue__JKI_lib_State_Machine.vi"("State(s) in Front (\"\")"="/* Post Error States", "State(s) in (\"\")"=w197) -> ("States Out"=w196:string)  [unwired: 13 in]
      }
      frame "Exit" {
        # "Do not put any code in this frame.\n(No errors that occur here will be handled.)"
        n89 = call <vilib>:"Add State(s) to Queue__JKI_lib_State_Machine.vi"("State(s) in (\"\")"=w202) -> ("States Out"=w201:string)  [unwired: 14 in]
      }
      frame "---------- Data ----------" {
        # "Do not put any code in this frame.\n(It is a separator no-op. You can make a copy of this frame to create a new Data frame)"
        n90 = call <vilib>:"Add State(s) to Queue__JKI_lib_State_Machine.vi"("State(s) in (\"\")"=w206) -> ("States Out"=w205:string)  [unwired: 14 in]
      }
      frame "Data: Load Image" {
        # "Do not put any code in this frame.\n(It is a separator no-op. You can make a copy of this frame to create a new Data frame)"
        n91 = Empty String/Path?(string/path="Path") -> (empty?=w209:bool)
        n92 = case shown="False" w209 {
          tunnel: w211 -> [w216 w228]
          tunnel: [w225 w228] -> w207
          tunnel: "Path" -> [w224 _]
          tunnel: [w218 _] -> w208
          frame False {
            w220 = T12 7 items=["Grayscale (U8)", "Grayscale (I16)", "Grayscale (SGL)", "Complex (CSG)", "RGB (U32)", "HSL (U32)", "RGB (U64)", "Grayscale (U16)"] ("Image Type")
            n93 = call "IMAQ Create"("Image Name"="img_in", "Image Type"=w220, "error in (no error)"=w216) -> ("New Image"=w222:T2, "error out"=w223:errorcluster)  [unwired: 2 in]
            n94 = call "IMAQ ReadFile 2"("File Path"=w224, "error in (no error)"=w223, "Image"=w222) -> ("error out"=w221:errorcluster, "Image Out"=w219:T2)  [unwired: 4 in, 3 out]
            n95 = call "IMAQ Clear Overlay"("error in (no error)"=w221, "Image"=w219) -> ("error out"=w227:errorcluster, "Image Out"=w218:T2)  [unwired: 8 in]
            "Image" <- w218
            n96 = property on="Image" class="ImageControl"(error in=w227, "ROI"=T6 {"Global Rectangle"=[], "Contours"=[]}) -> (error out=w225:errorcluster)  [unwired: 1 in, 1 out]
          }
          frame True {
          }
        }
        n97 = Bundle By Name(cluster=w213, "Image Out"=w208) -> (w212:T1)
        n98 = call <vilib>:"Add State(s) to Queue__JKI_lib_State_Machine.vi"("State(s) in (\"\")"=w215) -> ("States Out"=w214:string)  [unwired: 14 in]
      }
      frame "Data: Set Image" {
        # "Do not put any code in this frame.\n(It is a separator no-op. You can make a copy of this frame to create a new Data frame)"
        n99 = Unbundle By Name(w233) -> ("img_array"=w232:T2[])
        n100 = Index Array(array=w232, index="Image") -> (element=w229:T2)
        n101 = Bundle By Name(cluster=w233, "Image Out"=w229) -> (w234:T1)
        n102 = call <vilib>:"Add State(s) to Queue__JKI_lib_State_Machine.vi"("State(s) in (\"\")"=w236) -> ("States Out"=w235:string)  [unwired: 14 in]
      }
      frame "Data: Show Img" {
        # "Do not put any code in this frame.\n(It is a separator no-op. You can make a copy of this frame to create a new Data frame)"
        n103 = Unbundle By Name(w237) -> ("Image Out"=w238:T2)
        n104 = local write "Image"(w238) -> ()
        n105 = call <vilib>:"Add State(s) to Queue__JKI_lib_State_Machine.vi"("State(s) in (\"\")"=w241) -> ("States Out"=w240:string)  [unwired: 14 in]
      }
      frame "Data: Initialize" {
        w249 = dbl[][] []  # Temps_Array
        w250 = dbl[] []  # Temps
        w251 = T2[] []  # img_array
        w245 = 0  # State
        w253 = T13 {"Current VI Reference"=refnum, "Close Panel on Exit?"=FALSE}  # Core
        # "Initialize the shift-register data, here.\n(data names are defined by what you wire into the bundle function)"
        n106 = call "TCam_Calibration_LoadSettings.vi"("error in (no error)"=w248) -> ("error out"=w247:errorcluster, "Fixpoint Area"=w243:dbl, "Scan Area"=w244:dbl, "Points"=w246:T14)  [unwired: 7 in]
        n107 = local write "Fixpoint Radius"(w243) -> ()
        n108 = local write "Well Radius"(w244) -> ()
        n109 = local write "State"(w245) -> ()
        n110 = Bundle(cluster=T1 {"Core"={"Current VI Reference"=refnum, "Close Panel on Exit?"=FALSE}, "Image Out"=refnum, "State"=0, "Points"={"Top Left"={"X"=0.0, "Y"=0.0}, "Top Right"={"X"=0.0, "Y"=0.0}, "Bottom Left"={"X"=0.0, "Y"=0.0}, "Bottom Right"={"X"=0.0, "Y"=0.0}, "x space 2"=0.0, "y space 2"=0.0, "x_space"=0.0, "y_space"=0.0, "Pixels"=[], "Fixpoint"={"X"=0.0, "Y"=0.0}}, "img_array"=[], "Temps"=[], "Temps_Array"=[], "Scan Area"=0.0, "Fixpoint Area"=0.0, "PCR Size"=0} ("output cluster"), "Core"=w253, "Image Out"=T2 refnum, "State"=w245, "Points"=w246, "img_array"=w251, "Temps"=w250, "Temps_Array"=w249) -> (w254:T1)  [unwired: 3 in]
        n111 = call <vilib>:"Add State(s) to Queue__JKI_lib_State_Machine.vi"("State(s) in (\"\")"=w256) -> ("States Out"=w255:string)  [unwired: 14 in]
      }
      frame "Data: Cleanup" {
        # "Cleanup any data and references, here.\n(this is called automatically, by the Macro: Exit)"
        n112 = Unbundle By Name(w286) -> ("Points.Top Left"=w268:T3, "Points.Top Right"=w267:T3, "Points.Bottom Left"=w266:T3, "Points.Bottom Right"=w265:T3, "Points.Fixpoint"=w261:T3, "Core.Current VI Reference"=w287:refnum<vi>)
        n113 = local read "Fixpoint Radius"() -> (w259:i32)
        n114 = local read "Well Radius"() -> (w264:u32)
        n115 = Unbundle By Name(T7 {"Core"={"Current VI Reference"=refnum, "Close Panel on Exit?"=FALSE, "Exit"=FALSE, "Initialized?"=FALSE}, "Connections"={"cDAQ Therm"={"Task"="", "Connected"=FALSE, "Active"=FALSE}, "cDAQ Voltage"={"Task"="", "Connected"=FALSE, "Active"=FALSE}, "cDAQ ID"="", "Camera"={"Session"="", "Connected"=FALSE, "Active"=FALSE, "Placeholder"=refnum}, "PSU"={"Port"="", "Connected"=FALSE, "Active"=FALSE}}, "Data Acquisition"={"Setup"={"Label"="", "Operator"="", "Notes"="", "TempGrad"=1.0, "TargetTemp"=1.0, "Sample Volume"=1.0}, "Camera"={"Image"=refnum, "Save Image"=refnum, "Image Frequency"=20, "Rectangle"={"Left"=0, "Top"=0, "Right"=0, "Bottom"=0, "Rotation"=0.0}, "Calibration"={"Top Left"={"X"=0.0, "Y"=0.0}, "Top Right"={"X"=0.0, "Y"=0.0}, "Bottom Left"={"X"=0.0, "Y"=0.0}, "Bottom Right"={"X"=0.0, "Y"=0.0}, "Fixpoint"={"X"=0.0, "Y"=0.0}, "Scan Area"=5.0, "Fixpoint Area"=0.0, "Well Pixels"=[], "Valid"=FALSE}, "FocusPos"=0, "Display Mapping"=10}, "Thermistor"={"Sample Size"=1, "Calibration"={"B0.100"=[], "R25"=[], "c"=[], "State"=[], "V_S"=5.0, "R_S"=100.0}, "Timing Mode"=14713}, "Partition"={"Data"=[], "Cell Label"="", "Cell Color"=0, "Height"=10, "Width"=16, "Grid"=[]}, "Queue"={"Size"=1, "Queue"=refnum}, "Sample Rate"=20, "Active"=FALSE, "Ready"=FALSE, "Graph Mode"=0}, "Control"={"Sample Rate"=1, "PID gains"={"proportional gain (Kc)"=1.0, "integral time (Ti, min)"=0.01, "derivative time (Td, min)"=0.0}}} ("Default values")) -> ("Data Acquisition.Camera.Calibration"=w257:T15)
        n116 = Bundle(cluster=w257, "Top Left"=w268, "Top Right"=w267, "Bottom Left"=w266, "Bottom Right"=w265, "Fixpoint"=w261, "Scan Area"=w264, "Fixpoint Area"=w259, "Well Pixels"=cluster{"X":i32, "Y":i32}[][] [], "Valid"=FALSE) -> (w269:T15)
        n117 = call <vilib>:"Application Directory.vi"() -> ("Application Directory"=w281:path)
        n118 = Path To String(path=w281) -> (string=w282:string)
        n119 = Concatenate Strings(w282, "\\TCam.ini" ("string")) -> (w279:string)
        n120 = String To Path(string=w279) -> (path=w278:path)
        n121 = call <vilib>:"Check if File or Folder Exists.vi"("error in (no error)"=w271, "path"=w278) -> ("error out"=w275:errorcluster, "file or folder exists?"=w277:bool, "dup path"=w276:path)  [unwired: 7 in]
        n122 = case shown="True" w277 {
          tunnel: w276 -> [w290 w294]
          tunnel: w275 -> [w292 w295]
          tunnel: [w291 w295] -> w274
          tunnel: [w290 w294] -> w273
          frame False {
            n123 = Open/Create/Replace File(file path (use dialog)=w290, error in=w292, operation (0:open)=T10."create") -> (error out=w291:errorcluster)  [unwired: 3 in, 2 out]
          }
          frame True {
          }
        }
        n124 = Flatten To XML(6:w269) -> (2:w272:string)
        n125 = call-poly <vilib>:"Write to XML File.vi"("error in (no error)"=w274, "XML Input"=w272, "XML File Path"=w273) -> ("error out"=w270:errorcluster)  [unwired: 6 in, 2 out]
        n126 = local read "Image"() -> (w260:T2)
        n127 = Close Reference(reference=w287, error in (no error)=w270) -> (error out=w284:errorcluster)
        n128 = call "IMAQ Dispose"("All Images? (No)"=FALSE, "Image"=w260, "error in (no error)"=w284) -> ("error out"=w283:errorcluster)  [unwired: 3 in]
        n129 = call <vilib>:"Add State(s) to Queue__JKI_lib_State_Machine.vi"("State(s) in (\"\")"=w289) -> ("States Out"=w288:string)  [unwired: 14 in]
      }
      frame "---------- UI ----------" {
        # "Do not put any code in this frame.\n(It is a separator no-op. You can make a copy of this frame to create a new UI frame)"
        n130 = call <vilib>:"Add State(s) to Queue__JKI_lib_State_Machine.vi"("State(s) in (\"\")"=w299) -> ("States Out"=w298:string)  [unwired: 14 in]
      }
      frame "UI: Initialize" {
        w300 = u32 0 items=["Grayscale", "Binary", "Gradient", "Rainbow", "Temperature", "User Defined", "Binary 16 Bit", "Gradient 16 Bit", "Rainbow 16 Bit", "Temperature 16 Bit", "User Defined 16 Bit"] ("Palette:Palette Type")
        w305 = T12 4 items=["Grayscale (U8)", "Grayscale (I16)", "Grayscale (SGL)", "Complex (CSG)", "RGB (U32)", "HSL (U32)", "RGB (U64)", "Grayscale (U16)"] ("Image Type")
        w313 = u32 1 items=["Zoom Tool"=8, "Selection Tool"=0, "Pan Tool"=9, "Point Tool"=1, "Line Tool"=2, "Rectangle Tool"=3, "Rotated Rectangle Tool"=12, "Polyline Tool"=10, "Polygon Tool"=5, "Freehand Tool"=11, "Closed Freehand Tool"=6, "Ellipse Tool"=4, "Annulus Tool"=7] ("Current ROI Tool")
        w314 = u32 15 items=["Default"=10, "Most Significant Bits"=11, "Full Dynamic"=12, "Downshift"=13, "Given Range"=14, "90% Dynamic"=15, "Given Percent Range"=16] ("16-bit Display Mapping:Conversion Method")
        # "Initialize the User Interface, here.\n(this is called automatically, by the Macro: Init)"
        n131 = call <vilib>:"Application Directory.vi"() -> ("Application Directory"=w309:path)
        n132 = Path To String(path=w309) -> (string=w311:string)
        n133 = call "IMAQ Create"("Image Name"="placeholder_img_TCC", "Image Type"=w305) -> ("New Image"=w308:T2)  [unwired: 3 in, 1 out]
        n134 = Concatenate Strings(w311, "\\camera_placeholder.png") -> (w310:string)
        n135 = String To Path(string=w310) -> (path=w312:path)
        n136 = call "IMAQ ReadFile 2"("Use File Path Image Type"=FALSE, "File Path"=w312, "Image"=w308) -> ("Image Out"=w303:T2)  [unwired: 4 in, 4 out]
        n137 = property on="Image" class="ImageControl"("16-bit Display Conversion Method"=w314) -> ()  [unwired: 2 in, 2 out]
        n138 = property on="Image" class="ImageControl"("Current ROI Tool"=w313, "Palette Type"=w300) -> ()  [unwired: 2 in, 2 out]
        n139 = local write "Display Mapping"(w314) -> ()
        n140 = local write "Image"(w303) -> ()
        n141 = local write "Path"(path "" ("Path")) -> ()
        n142 = property on="Image" class="ImageControl"("Zoom to Fit Mode"=TRUE) -> ()  [unwired: 2 in, 2 out]
        n143 = call <vilib>:"Add State(s) to Queue__JKI_lib_State_Machine.vi"("State(s) in Front (\"\")"="UI: Tutorial\n// UI: Progress >> Hide" ("State(s) in Front (\"\")"), "State(s) in (\"\")"=w319) -> ("States Out"=w318:string)  [unwired: 13 in]
      }
      frame "UI: Tutorial" {
        # "Initialize the User Interface, here.\n(this is called automatically, by the Macro: Init)"
        n144 = local read "State"() -> (w334:i32)
        n145 = case shown="2" w334 {
          tunnel: ["Load Calibration Image." "Select a Display Mapping that shows a clear image.\n\nSelect correct PCR size." w353 w371 w378 w385 "Select Well Radius so the center of each well is covered.\n\nGo to previous steps to adjust positions. Press done once satisfied."] -> w333
          tunnel: [_ _ _ _ _ _ w390] -> w332
          tunnel: [_ _ _ _ _ _ w390] -> w331
          tunnel: [_ w346 _ _ _ _ _] -> w330
          tunnel: [_ w346 _ _ _ _ _] -> w329
          tunnel: [w338 w346 w354 w368 w375 w382 _] -> w328
          tunnel: [_ w346 w360 w366 w372 w380 w390] -> w327
          tunnel: [TRUE _ _ _ _ _ _] -> w326
          tunnel: [_ _ w351 _ _ _ _] -> w325
          tunnel: w324 -> [_ _ w363 w369 w376 w383 _]
          tunnel: ["Step: 1/7" "Step: 2/7" "Step: 3/7" "Step: 4/7" "Step: 5/7" "Step: 6/7" "Step: 7/7"] -> w323
          tunnel: [_ _ _ _ _ _ w388] -> w322
          tunnel: [_ TRUE w360 w366 w372 w380 TRUE] -> w321
          tunnel: [_ 0 ("t") w357 3 ("t") 4 ("t") 5 ("t") 6 ("t")] -> w320
          frame 0, Default {
            n146 = local read "Path"() -> (w340:path)
            n147 = Empty String/Path?(string/path=w340) -> (empty?=w339:bool)
            n148 = Not(x=w339) -> (.not. x?=w338:bool)
          }
          frame 1 {
            w346 = TRUE
          }
          frame 2 {
            w360 = TRUE
            w364 = "Select Fix Point Cavity (Left Click) as shown (zoom with Mouse Wheel).\n\n"  # Select Fix Point Cavity (Left Click) as shown (zoom with Mouse Wheel).
            n149 = Unbundle By Name(w363) -> ("Points.Fixpoint.X"=w362:sgl)
            n150 = local read "Fixpoint Radius"() -> (w356:i32)
            n151 = Not Equal To 0?(x=w362) -> (x != 0?=w351:bool)
            n152 = Not Equal To 0?(x=w356) -> (x != 0?=w355:bool)
            n153 = And(x=w355, y=w351) -> (x .and. y?=w354:bool)
            n154 = Select(t="Set Fixpoint Radius so the cavity is appropriately filled as shown. ", s=w351, f="") -> (s? t:f=w352:string)
            n155 = Select(t=2, s=w351, f=1) -> (s? t:f=w357:i32)
            n156 = Concatenate Strings(w364, w352) -> (w353:string)
          }
          frame 3 {
            w366 = TRUE
            w371 = "Select Top Left corner of PCR plate as shown."  # Select Top Left corner of PCR plate as shown.
            n157 = Unbundle By Name(w369) -> ("Points.Top Left.X"=w370:sgl)
            n158 = Not Equal To 0?(x=w370) -> (x != 0?=w368:bool)
          }
          frame 4 {
            w372 = TRUE
            w378 = "Select Top Right corner of PCR plate as shown."  # Select Top Right corner of PCR plate as shown.
            n159 = Unbundle By Name(w376) -> ("Points.Top Right.X"=w377:sgl)
            n160 = Not Equal To 0?(x=w377) -> (x != 0?=w375:bool)
          }
          frame 5 {
            w380 = TRUE
            w385 = "Select Bottom Left corner of PCR plate as shown."  # Select Bottom Left corner of PCR plate as shown.
            n161 = Unbundle By Name(w383) -> ("Points.Bottom Left.X"=w384:sgl)
            n162 = Not Equal To 0?(x=w384) -> (x != 0?=w382:bool)
          }
          frame 6 {
            w390 = TRUE
            n163 = local read "Well Radius"() -> (w389:u32)
            n164 = Not Equal To 0?(x=w389) -> (x != 0?=w388:bool)
          }
        }
        "Tutorial" <- w333
        "Step" <- w323
        "Pict Ring" <- w320
        n165 = property on="Fixpoint Radius" class="DigNum (strict)"("Visible"=w325) -> ()  [unwired: 2 in, 2 out]
        n166 = property on="Path" class="Path"("Visible"=w326) -> ()  [unwired: 2 in, 2 out]
        n167 = property on="Well Radius" class="DigNum (strict)"("Visible"=w332) -> ()  [unwired: 2 in, 2 out]
        n168 = property on="Show All Points" class="Bool (strict)"("Visible"=w331) -> ()  [unwired: 2 in, 2 out]
        n169 = property on="Display Mapping" class="Ring (strict)"("Visible"=w330) -> ()  [unwired: 2 in, 2 out]
        n170 = property on="PCR Size" class="Ring (strict)"("Visible"=w329) -> ()  [unwired: 2 in, 2 out]
        n171 = property on="Next" class="Bool"("Visible"=w328) -> ()  [unwired: 2 in, 2 out]
        n172 = property on="Previous" class="Bool"("Visible"=w327) -> ()  [unwired: 2 in, 2 out]
        n173 = property on="Done" class="Bool"("Visible"=w322) -> ()  [unwired: 2 in, 2 out]
        n174 = property on="Pict Ring" class="Ring (strict)"("Visible"=w321) -> ()  [unwired: 2 in, 2 out]
        n175 = call <vilib>:"Add State(s) to Queue__JKI_lib_State_Machine.vi"("State(s) in (\"\")"=w337) -> ("States Out"=w336:string)  [unwired: 14 in]
      }
      frame "UI: Cursor Set" {
        # "Argument"
        # "Set and Unset Cursor Busy.\n(Usage: \"UI: Cursor Set >> Busy|Idle\")"
        n176 = case shown="\"Busy\"" w393 {
          tunnel: w395 -> [w400 w402]
          tunnel: [w399 w401] -> w394
          frame "Idle", Default {
            n177 = call <vilib>:"Unset Busy.vi"("error in (no error)"=w400) -> ("error out"=w399:errorcluster)  [unwired: 10 in]
          }
          frame "Busy" {
            n178 = call <vilib>:"Set Busy.vi"("error in (no error)"=w402) -> ("error out"=w401:errorcluster)  [unwired: 9 in, 1 out]
          }
        }
        n179 = call <vilib>:"Add State(s) to Queue__JKI_lib_State_Machine.vi"("State(s) in (\"\")"=w398) -> ("States Out"=w397:string)  [unwired: 14 in]
      }
      frame "UI: Front Panel State" {
        # "Argument"
        # "Set Front Panel Open or Closed\n(Usage: \"UI: Front Panel State >> Open|Close\")"
        n180 = Unbundle By Name(w405) -> ("Core.Current VI Reference"=w404:refnum<vi>)
        n181 = case shown="\"Close\", \"Closed\"" w403 {
          tunnel: w407 -> [w415 w430 w441 w454 w467]
          tunnel: [w417 w431 w443 w456 w469] -> w406
          tunnel: w404 -> [w416 w428 w442 w455 w468]
          frame "Open", "Standard", Default {
            w410 = T4."Standard" ("State")
            n182 = property class="VI"(reference=w416, error in=w415) -> (reference out=w413:refnum<vi>, error out=w414:errorcluster, "FP.State"=w412:T4)
            n183 = Not Equal?(x=w412, y=w410) -> (x != y?=w411:bool)
            n184 = case shown="True" w411 {
              tunnel: [w421 w423] -> w417
              tunnel: w414 -> [w420 w423]
              tunnel: w413 -> [w419 _]
              tunnel: w410 -> [w418 _]
              frame True {
                n185 = invoke class="VI" method="FP.Open"(reference=w419, error in=w420, "Activate"=TRUE, "State"=w418) -> (error out=w421:errorcluster)  [unwired: 1 in, 4 out]
              }
              frame False {
              }
            }
          }
          frame "Close", "Closed" {
            n186 = property class="VI"(reference=w428, error in=w430) -> (reference out=w427:refnum<vi>, error out=w429:errorcluster, "FP.State"=w425:T4)
            n187 = Not Equal?(x=w425, y=T4."Closed" ("Front Panel Window:State")) -> (x != y?=w424:bool)
            n188 = case shown="True" w424 {
              tunnel: [w432 w435] -> w431
              tunnel: w429 -> [w432 w434]
              tunnel: w427 -> [_ w433]
              frame False {
              }
              frame True {
                n189 = invoke class="VI" method="FP.Close"(reference=w433, error in=w434) -> (error out=w435:errorcluster)  [unwired: 1 in, 2 out]
              }
            }
          }
          frame "Hidden", "Hide" {
            w436 = T4."Hidden" ("State")
            n190 = property class="VI"(reference=w442, error in=w441) -> (reference out=w439:refnum<vi>, error out=w440:errorcluster, "FP.State"=w438:T4)
            n191 = Not Equal?(x=w438, y=w436) -> (x != y?=w437:bool)
            n192 = case shown="True" w437 {
              tunnel: [w447 w448] -> w443
              tunnel: w440 -> [w446 w448]
              tunnel: w439 -> [w445 _]
              tunnel: w436 -> [w444 _]
              frame True {
                n193 = invoke class="VI" method="FP.Open"(reference=w445, error in=w446, "State"=w444) -> (error out=w447:errorcluster)  [unwired: 2 in, 4 out]
              }
              frame False {
              }
            }
          }
          frame "Minimize", "Minimized" {
            w449 = T4."Minimized" ("State")
            n194 = property class="VI"(reference=w455, error in=w454) -> (reference out=w452:refnum<vi>, error out=w453:errorcluster, "FP.State"=w451:T4)
            n195 = Not Equal?(x=w451, y=w449) -> (x != y?=w450:bool)
            n196 = case shown="True" w450 {
              tunnel: [w460 w461] -> w456
              tunnel: w453 -> [w459 w461]
              tunnel: w452 -> [w458 _]
              tunnel: w449 -> [w457 _]
              frame True {
                n197 = invoke class="VI" method="FP.Open"(reference=w458, error in=w459, "State"=w457) -> (error out=w460:errorcluster)  [unwired: 2 in, 4 out]
              }
              frame False {
              }
            }
          }
          frame "Maximize", "Maximized" {
            w462 = T4."Maximized" ("State")
            n198 = property class="VI"(reference=w468, error in=w467) -> (reference out=w465:refnum<vi>, error out=w466:errorcluster, "FP.State"=w464:T4)
            n199 = Not Equal?(x=w464, y=w462) -> (x != y?=w463:bool)
            n200 = case shown="True" w463 {
              tunnel: [w473 w474] -> w469
              tunnel: w466 -> [w472 w474]
              tunnel: w465 -> [w471 _]
              tunnel: w462 -> [w470 _]
              frame True {
                n201 = invoke class="VI" method="FP.Open"(reference=w471, error in=w472, "State"=w470) -> (error out=w473:errorcluster)  [unwired: 2 in, 4 out]
              }
              frame False {
              }
            }
          }
        }
        n202 = call <vilib>:"Add State(s) to Queue__JKI_lib_State_Machine.vi"("State(s) in (\"\")"=w409) -> ("States Out"=w408:string)  [unwired: 14 in]
      }
      frame "---------- Macro ----------" {
        # "Do not put any code in this frame.\n(It is a separator no-op. You can make a copy of this frame to create a new Macro frame)"
        n203 = call <vilib>:"Add State(s) to Queue__JKI_lib_State_Machine.vi"("State(s) in (\"\")"=w478) -> ("States Out"=w477:string)  [unwired: 14 in]
      }
      frame "Macro: Initialize" {
        w479 = "// UI: Cursor Set >> Busy\nData: Initialize\nInitialize Core Data\nUI: Initialize\nUI: Front Panel State >> Show\nUI: Tutorial\n// Image: Draw\n// UI: Cursor Set >> Idle"  # // UI: Cursor Set >> Busy Data: Initialize Initialize Core Data UI: Initialize UI: Front Panel State >> Show UI: Tutorial // Image: Draw // UI: Cursor Set >> Idle
        # "Initialization Macro\n(This is called once, when the VI starts)"
        n204 = call <vilib>:"Add State(s) to Queue__JKI_lib_State_Machine.vi"("State(s) in Front (\"\")"=w479, "State(s) in (\"\")"=w483) -> ("States Out"=w482:string)  [unwired: 13 in]
      }
      frame "Macro: Exit" {
        # "Exit Macro\n(This is called once, when the VI exits)"
        n205 = Unbundle By Name(w491) -> ("Core.Close Panel on Exit?"=w490:bool)
        n206 = Select(t="UI: Front Panel State >> Close", s=w490, f="") -> (s? t:f=w487:string)
        n207 = call <vilib>:"Add State(s) to Queue__JKI_lib_State_Machine.vi"("State(s) in Front (\"\")"="Data: Cleanup" ("State(s) in Front (\"\")"), "State(s) in (\"\")"=w487, "State(s) at Back (\"\")"="Exit") -> ("States Out"=w485:string)  [unwired: 12 in]
        n208 = call <vilib>:"Add State(s) to Queue__JKI_lib_State_Machine.vi"("State(s) in Front (\"\")"=w485, "State(s) in (\"\")"=w494) -> ("States Out"=w493:string)  [unwired: 13 in]
      }
      frame "---------- Image ----------" {
        # "Template Separator\n(You can make a copy of, or modify, this frame)"
        n209 = call <vilib>:"Add State(s) to Queue__JKI_lib_State_Machine.vi"("State(s) in (\"\")"=w498) -> ("States Out"=w497:string)  [unwired: 14 in]
      }
      frame "Image: Draw" {
        # "Template Separator\n(You can make a copy of, or modify, this frame)"
        n210 = call <vilib>:"Add State(s) to Queue__JKI_lib_State_Machine.vi"("State(s) in Front (\"\")"="UI: Cursor Set >> Busy\nImage: Clear ROI\nImage: Set ROI\nImage: Draw Fixedpoint\nImage: Calculate BR\nImage: Calculate y space\nImage: Calculate x space\nImage: Calculate Positions\nImage: Drawlines\nImage: Draw Points\nUI: Cursor Set >> Idle" ("State(s) in Front (\"\")"), "State(s) in (\"\")"=w503) -> ("States Out"=w502:string)  [unwired: 13 in]
      }
      frame "Image: Redraw" {
        # "Template Separator\n(You can make a copy of, or modify, this frame)"
        n211 = call <vilib>:"Add State(s) to Queue__JKI_lib_State_Machine.vi"("State(s) in Front (\"\")"="UI: Cursor Set >> Busy\nImage: Clear ROI\nImage: Drawlines\nImage: Draw Points\nImage: Calculate Temps\nUI: Cursor Set >> Idle" ("State(s) in Front (\"\")"), "State(s) in (\"\")"=w508) -> ("States Out"=w507:string)  [unwired: 13 in]
      }
      frame "Image: Drawlines" {
        # "Template Separator\n(You can make a copy of, or modify, this frame)"
        n212 = Unbundle By Name(w509) -> ("Points.Top Left.X"=w525:sgl, "Points.Top Right.X"=w524:sgl, "Points.Bottom Left.X"=w523:sgl, "Points.Bottom Right.X"=w522:sgl)
        n213 = Equal To 0?(x=w522) -> (x = 0?=w512:bool)
        n214 = Equal To 0?(x=w523) -> (x = 0?=w511:bool)
        n215 = Or(x=w511, y=w512) -> (x .or. y?=w510:bool)
        n216 = Equal To 0?(x=w525) -> (x = 0?=w521:bool)
        n217 = Equal To 0?(x=w524) -> (x = 0?=w520:bool)
        n218 = Select(t="", s=w511, f="Image: Draw Line >> TL_BL\n") -> (s? t:f=w517:string)
        n219 = Select(t="", s=w510, f="Image: Draw Line >> TR_BR\nImage: Draw Line >> BL_BR\nImage: Draw Line >> Vertical\nImage: Draw Line >> Horizontal") -> (s? t:f=w514:string)
        n220 = case shown="False" w521 {
          tunnel: w520 -> [w532 _]
          tunnel: w517 -> [w531 _]
          tunnel: w514 -> [w530 _]
          tunnel: [w529 _] -> w513
          frame False {
            n221 = case shown="False" w532 {
              tunnel: w531 -> [w535 _]
              tunnel: w530 -> [w534 _]
              tunnel: [w533 _] -> w529
              frame False {
                n222 = Concatenate Strings("Image: Draw Line >> TL_TR\n", w535, w534) -> (w533:string)
              }
              frame True {
              }
            }
          }
          frame True {
          }
        }
        n223 = call <vilib>:"Add State(s) to Queue__JKI_lib_State_Machine.vi"("State(s) in Front (\"\")"=w513, "State(s) in (\"\")"=w528) -> ("States Out"=w527:string)  [unwired: 13 in]
      }
      frame "Image: Draw Fixedpoint" {
        # "Template Separator\n(You can make a copy of, or modify, this frame)"
        n224 = Unbundle By Name(w543) -> ("Image Out"=w540:T2, "Points.Fixpoint"=w542:T3)
        n225 = Build Array(w542) -> (w541:T3[])
        n226 = call "TCam_CenterArray.vi"("Size"="Fixpoint Radius", "Point Array"=w541, "Image in"=w540) -> ("Image"=w539:T2)  [unwired: 3 in, 1 out]
        n227 = local write "Image"(w539) -> ()
        n228 = call <vilib>:"Add State(s) to Queue__JKI_lib_State_Machine.vi"("State(s) in (\"\")"=w545) -> ("States Out"=w544:string)  [unwired: 14 in]
      }
      frame "Image: Clear ROI" {
        # "Your code here.\n(You can make a copy of, or modify, this frame)"
        n229 = Unbundle By Name(w549) -> ("Image Out"=w548:T2)
        n230 = call "IMAQ Clear Overlay"("error in (no error)"=w547, "Image"=w548) -> ("error out"=w546:errorcluster)  [unwired: 8 in, 1 out]
        n231 = call <vilib>:"Add State(s) to Queue__JKI_lib_State_Machine.vi"("State(s) in (\"\")"=w551) -> ("States Out"=w550:string)  [unwired: 14 in]
      }
      frame "Image: Calculate x space" {
        # "Your code here.\n(You can make a copy of, or modify, this frame)"
        n232 = Unbundle By Name(w560) -> ("Points.Top Left"=w566:T3, "Points.Top Right"=w565:T3)
        n233 = case shown="1" "PCR Size" {
          tunnel: [24 12] -> w552
          frame 0, Default {
          }
          frame 1 {
          }
        }
        n234 = Unbundle(w565) -> ("X"=w564:sgl, "Y"=w562:sgl)
        n235 = Unbundle(w566) -> ("X"=w563:sgl, "Y"=w561:sgl)
        n236 = Subtract(x=w564, y=w563) -> (x-y=w557:sgl)
        n237 = Decrement(x=w552) -> (x-1=w556:i32)
        n238 = Subtract(x=w562, y=w561) -> (x-y=w555:sgl)
        n239 = Divide(x=w557, y=w556) -> (x/y=w558:sgl)
        n240 = Divide(x=w555, y=w556) -> (x/y=w554:sgl)
        n241 = Bundle By Name(cluster=w560, "Points.x_space"=w558, "Points.y_space"=w554) -> (w559:T1)
        n242 = call <vilib>:"Add State(s) to Queue__JKI_lib_State_Machine.vi"("State(s) in (\"\")"=w569) -> ("States Out"=w568:string)  [unwired: 14 in]
      }
      frame "Image: Calculate BR" {
        # "Your code here.\n(You can make a copy of, or modify, this frame)"
        n243 = Unbundle By Name(w580) -> ("Points.Top Left"=w586:T3, "Points.Top Right"=w585:T3, "Points.Bottom Left"=w578:T3)
        n244 = Unbundle(w586) -> ("X"=w583:sgl, "Y"=w581:sgl)
        n245 = Unbundle(w585) -> ("X"=w584:sgl, "Y"=w582:sgl)
        n246 = Unbundle(w578) -> ("X"=w577:sgl, "Y"=w575:sgl)
        n247 = Subtract(x=w584, y=w583) -> (x-y=w576:sgl)
        n248 = Subtract(x=w582, y=w581) -> (x-y=w574:sgl)
        n249 = Add(x=w577, y=w576) -> (x+y=w572:sgl)
        n250 = Add(x=w574, y=w575) -> (x+y=w573:sgl)
        n251 = Bundle By Name(cluster=w580, "Points.Bottom Right.X"=w572, "Points.Bottom Right.Y"=w573) -> (w579:T1)
        n252 = call <vilib>:"Add State(s) to Queue__JKI_lib_State_Machine.vi"("State(s) in (\"\")"=w589) -> ("States Out"=w588:string)  [unwired: 14 in]
      }
      frame "Image: Calculate y space" {
        # "Your code here.\n(You can make a copy of, or modify, this frame)"
        n253 = local read "PCR Size"() -> (w591:u16)
        n254 = Unbundle By Name(w598) -> ("Points.Top Left"=w604:T3, "Points.Bottom Left"=w603:T3)
        n255 = case shown="1" w591 {
          tunnel: [16 8] -> w590
          frame 0, Default {
          }
          frame 1 {
          }
        }
        n256 = Unbundle(w603) -> ("X"=w602:sgl, "Y"=w600:sgl)
        n257 = Unbundle(w604) -> ("X"=w601:sgl, "Y"=w599:sgl)
        n258 = Subtract(x=w602, y=w601) -> (x-y=w595:sgl)
        n259 = Decrement(x=w590) -> (x-1=w594:i32)
        n260 = Subtract(x=w600, y=w599) -> (x-y=w593:sgl)
        n261 = Divide(x=w595, y=w594) -> (x/y=w596:sgl)
        n262 = Divide(x=w593, y=w594) -> (x/y=w592:sgl)
        n263 = Bundle By Name(cluster=w598, "Points.x space 2"=w596, "Points.y space 2"=w592) -> (w597:T1)
        n264 = call <vilib>:"Add State(s) to Queue__JKI_lib_State_Machine.vi"("State(s) in (\"\")"=w607) -> ("States Out"=w606:string)  [unwired: 14 in]
      }
      frame "Image: Set ROI" {
        # "Your code here.\n(You can make a copy of, or modify, this frame)"
        n265 = Unbundle By Name(w616) -> ("State"=w614:i32)
        n266 = case shown="2..5" w614 {
          tunnel: w614 -> [_ w628]
          tunnel: w616 -> [_ w626]
          tunnel: w615 -> [w621 w625]
          tunnel: [w621 w624] -> w613
          tunnel: [T11 {"Global Rectangle"=[], "Contours"=[]} ("ROI Descriptor") w623] -> w612
          tunnel: [w619 w622] -> w610
          frame 0, Default {
            w619 = u32 0 items=["Zoom Tool"=8, "Selection Tool"=0, "Pan Tool"=9, "Point Tool"=1, "Line Tool"=2, "Rectangle Tool"=3, "Rotated Rectangle Tool"=12, "Polyline Tool"=10, "Polygon Tool"=5, "Freehand Tool"=11, "Closed Freehand Tool"=6, "Ellipse Tool"=4, "Annulus Tool"=7] ("Current ROI Tool")
          }
          frame 2..5 {
            w622 = u32 1 items=["Zoom Tool"=8, "Selection Tool"=0, "Pan Tool"=9, "Point Tool"=1, "Line Tool"=2, "Rectangle Tool"=3, "Rotated Rectangle Tool"=12, "Polyline Tool"=10, "Polygon Tool"=5, "Freehand Tool"=11, "Closed Freehand Tool"=6, "Ellipse Tool"=4, "Annulus Tool"=7] ("Current ROI Tool")
            n267 = case shown="5" w628 {
              tunnel: [w630 w632 w634 w636] -> w627
              tunnel: w626 -> [w629 w631 w633 w635]
              frame 2, Default {
                n268 = Unbundle By Name(w629) -> ("Points.Fixpoint"=w630:T3)
              }
              frame 3 {
                n269 = Unbundle By Name(w631) -> ("Points.Top Left"=w632:T3)
              }
              frame 4 {
                n270 = Unbundle By Name(w633) -> ("Points.Top Right"=w634:T3)
              }
              frame 5 {
                n271 = Unbundle By Name(w635) -> ("Points.Bottom Left"=w636:T3)
              }
            }
            n272 = call "IMAQ Convert Point to ROI"("error in (no error)"=w625, "Point"=w627) -> ("error out"=w624:errorcluster, "ROI Descriptor"=w623:T11)  [unwired: 7 in]
          }
        }
        n273 = property on="Image" class="ImageControl"("Current ROI Tool"=w610) -> ()  [unwired: 2 in, 2 out]
        n274 = property on="Image" class="ImageControl"(error in=w613, "ROI"=w612) -> (error out=w611:errorcluster)  [unwired: 1 in, 1 out]
        n275 = call <vilib>:"Add State(s) to Queue__JKI_lib_State_Machine.vi"("State(s) in (\"\")"=w618) -> ("States Out"=w617:string)  [unwired: 14 in]
      }
      frame "Image: Draw Line" {
        w637 = u32 1  # Width_Minor
        w638 = u32 2  # Width
        # "Your code here.\n(You can make a copy of, or modify, this frame)"
        n276 = Unbundle By Name(w642) -> ("Image Out"=w643:T2)
        n277 = case shown="\"Vertical\"" w644 {
          tunnel: w643 -> [w648 w656 w665 w672 w678 w683 w692]
          tunnel: w642 -> [_ w657 w666 w668 w674 w687 w696]
          tunnel: [w648 w651 w664 w671 w677 w679 w688] -> w641
          tunnel: w640 -> [w647 w655 w663 w670 w676 w681 w691]
          tunnel: [w647 w650 w662 w669 w675 w680 w690] -> w639
          tunnel: w638 -> [_ w649 w658 _ _ w682 w689]
          tunnel: w637 -> [_ _ _ w667 w673 _ _]
          frame "False", Default {
          }
          frame "TL_TR" {
            n278 = Unbundle By Name(w657) -> ("Points.Top Left"=w654:T3, "Points.Top Right"=w653:T3)
            n279 = Build Array(w654, w653) -> (w652:T3[])
            n280 = call "IMAQ Overlay Multiple Lines 2"("Image"=w656, "Line End Points"=w652, "error in (no error)"=w655, "Width"=w649) -> ("Image Out"=w651:T2, "error out"=w650:errorcluster)  [unwired: 10 in]
          }
          frame "TL_BL" {
            n281 = Unbundle By Name(w666) -> ("Points.Top Left"=w661:T3, "Points.Bottom Left"=w660:T3)
            n282 = Build Array(w661, w660) -> (w659:T3[])
            n283 = call "IMAQ Overlay Multiple Lines 2"("Image"=w665, "Line End Points"=w659, "error in (no error)"=w663, "Width"=w658) -> ("Image Out"=w664:T2, "error out"=w662:errorcluster)  [unwired: 10 in]
          }
          frame "Vertical" {
            n284 = call "TCam_VerticalLines.vi"("Width"=w667, "error in (no error)"=w670, "Cluster"=w668, "Refnum in"=w672) -> ("error out"=w669:errorcluster, "Refnum out"=w671:T2)  [unwired: 6 in]
          }
          frame "Horizontal" {
            n285 = call "TCam_HorizontalLines.vi"("Width"=w673, "error in (no error)"=w676, "Cluster"=w674, "Refnum in"=w678) -> ("error out"=w675:errorcluster, "Refnum out"=w677:T2)  [unwired: 6 in]
          }
          frame "TR_BR" {
            n286 = Unbundle By Name(w687) -> ("Points.Top Right"=w686:T3, "Points.Bottom Right"=w685:T3)
            n287 = Build Array(w686, w685) -> (w684:T3[])
            n288 = call "IMAQ Overlay Multiple Lines 2"("Image"=w683, "Line End Points"=w684, "error in (no error)"=w681, "Width"=w682) -> ("Image Out"=w679:T2, "error out"=w680:errorcluster)  [unwired: 10 in]
          }
          frame "BL_BR" {
            n289 = Unbundle By Name(w696) -> ("Points.Bottom Left"=w695:T3, "Points.Bottom Right"=w694:T3)
            n290 = Build Array(w695, w694) -> (w693:T3[])
            n291 = call "IMAQ Overlay Multiple Lines 2"("Image"=w692, "Line End Points"=w693, "error in (no error)"=w691, "Width"=w689) -> ("Image Out"=w688:T2, "error out"=w690:errorcluster)  [unwired: 10 in]
          }
        }
        n292 = local write "Image"(w641) -> ()
        n293 = call <vilib>:"Add State(s) to Queue__JKI_lib_State_Machine.vi"("State(s) in (\"\")"=w646) -> ("States Out"=w645:string)  [unwired: 14 in]
      }
      frame "Image: Draw Points" {
        # "Your code here.\n(You can make a copy of, or modify, this frame)"
        n294 = Unbundle By Name(w698) -> ("Points.Top Left.X"=w707:sgl, "Points.Top Right.X"=w706:sgl, "Points.Bottom Left.X"=w705:sgl, "Points.Bottom Right.X"=w704:sgl)
        n295 = Equal To 0?(x=w707) -> (x = 0?=w703:bool)
        n296 = Equal To 0?(x=w706) -> (x = 0?=w702:bool)
        n297 = Equal To 0?(x=w705) -> (x = 0?=w701:bool)
        n298 = Equal To 0?(x=w704) -> (x = 0?=w700:bool)
        n299 = Unbundle By Name(w698) -> ("Image Out"=w709:T2)
        n300 = Compound Arithmetic op=OR(w703, w702, w701, w700) -> (w699:bool)
        n301 = case shown="False" w699 {
          tunnel: w709 -> [w719 _]
          tunnel: w698 -> [w714 w720]
          tunnel: [w712 w720] -> w697
          frame False {
            n302 = local read "Points"() -> (w718:T3[])
            n303 = call "TCam_CenterArray.vi"("draw all?"="Show All Points", "Size"="Well Radius", "Point Array"=w718, "Image in"=w719) -> ("Array"=w713:cluster{"X":i32, "Y":i32}[][], "Image"=w716:T2)  [unwired: 2 in]
            n304 = local write "Image"(w716) -> ()
            n305 = Bundle By Name(cluster=w714, "Points.Pixels"=w713) -> (w712:T1)
          }
          frame True {
          }
        }
        n306 = call <vilib>:"Add State(s) to Queue__JKI_lib_State_Machine.vi"("State(s) in (\"\")"=w711) -> ("States Out"=w710:string)  [unwired: 14 in]
      }
      frame "Image: Calculate Positions" {
        # "Your code here.\n(You can make a copy of, or modify, this frame)"
        n307 = Unbundle By Name(w722) -> ("Points.Top Left.X"=w730:sgl, "Points.Top Right.X"=w729:sgl, "Points.Bottom Left.X"=w728:sgl, "Points.Bottom Right.X"=w727:sgl)
        n308 = Equal To 0?(x=w730) -> (x = 0?=w726:bool)
        n309 = Equal To 0?(x=w729) -> (x = 0?=w725:bool)
        n310 = Equal To 0?(x=w728) -> (x = 0?=w724:bool)
        n311 = Equal To 0?(x=w727) -> (x = 0?=w723:bool)
        n312 = Compound Arithmetic op=OR(w726, w725, w724, w723) -> (w721:bool)
        n313 = case shown="False" w721 {
          tunnel: w722 -> [w734 _]
          frame False {
            n314 = local read "PCR Size"() -> (w735:u16)
            n315 = call "TCam_PointCalculator.vi"("Cluster"=w734, "Size"=w735) -> ("Points"=→"Points":T3[])  [unwired: 9 in]
          }
          frame True {
          }
        }
        n316 = call <vilib>:"Add State(s) to Queue__JKI_lib_State_Machine.vi"("State(s) in (\"\")"=w733) -> ("States Out"=w732:string)  [unwired: 14 in]
      }
    }
  }
  "State out" <- "Data: Load Thermal Calibration"
